vi "Dashboard custom_bartender&global&gripper&camera3.vi"() -> ()   [LabVIEW 2017]
uses:
  C:/Users/IMR Lab/Documents/LabVIEW Data/UniversalRobotsSDK_LABView/LabVIEW/Examples/LabVIEW10/UnderAutomation.UniversalRobots.dll
  UnderAutomation.UniversalRobots.dll
  Global 1.vi
panel:
  out "3rd Order":bool
  out "2nd Order":bool
  out "1st Order":bool
  out "Rx":dbl
  out "Rz":dbl
  out "Ry":dbl
  out "Enabled":bool
  out "Port":i32
  in  "Move to particular posture":bool
  in  "Move to Zero position":bool
  out "Connected":bool
  in  "Robot IP(192.168.112.182)":string
  out "Connect error":errorcluster
  in  "Power on\nRelease brake":bool
  in  "Power off":bool
  in  "Connect":bool
  in  "Send script":bool
  in  "Script to execute":string
  out "Powered on":bool
  out "X":dbl
  out "Y":dbl
  out "Z":dbl
  out "License state":string
  # "e"
  # "movej( get_inverse_kin(p[0.3138, 0.0814, 0.1647, 0.4226, -2.3876, -2.3851]),  a=0.5, v=0.25, t=0, r=0)"
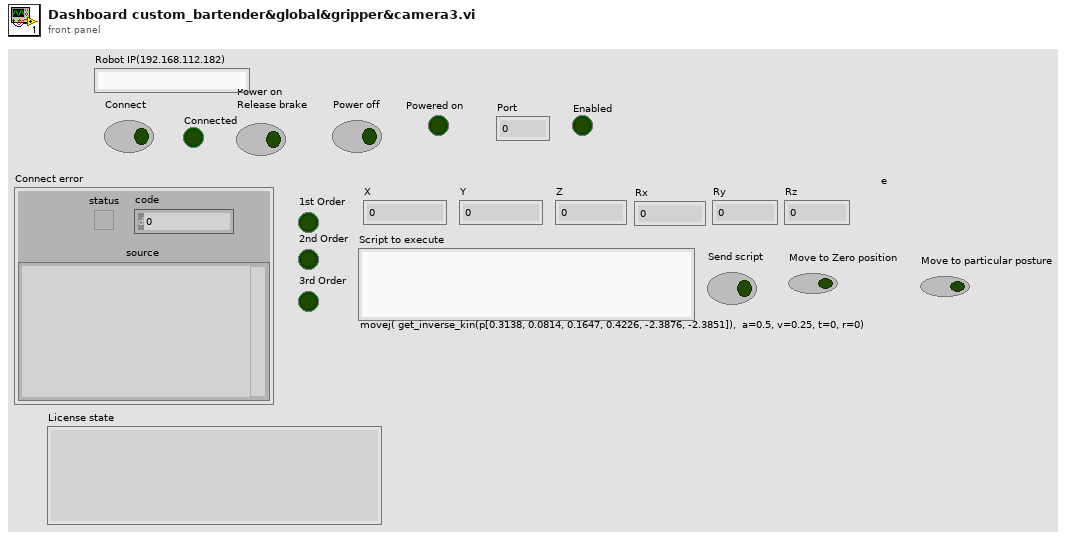
[diagram p1: front panel]
types:
  T1 = enum16{"Standard", "Buffered", "CRLF", "Immediate"}
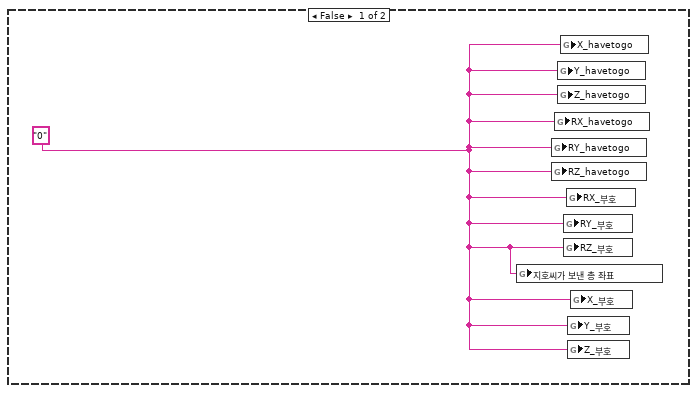
[diagram p2: hidden frame]
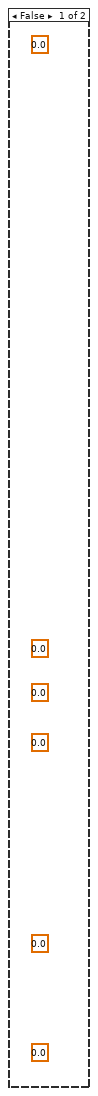
[diagram p3: hidden frame]
diagram:
  w2 = ""
  # "미니콜라 따르는 자세"
  # "술잔 중간지점 가는 자세"
  # "짐빔에서 토닉이동 준비 자세"
  # "술잔 따르는 자세2"
  # "술잔 위로 가는 자세2"
  # "토닉워터 뺴는 자세"
  # "토닉워 들어올리는 자세"
  # "토닉워터 가는 자세"
  # "토닉워터 보는 자세"
  # "짐빔 들어올리는 자세"
  # "짐빔로 가는 자세"
  # "짐빔 보는 자세"
  # "콜라 뺴는 자세"
  # "콜라 들어올리는 자세"
  # "콜라로 가는 자세"
  # "콜라 보는 자세"
  # "술잔 따르는 자세"
  # "술잔 위로 가는 자세"
  # "잭다니엘 들어올리는 자세"
  # "잭다니엘 위치로 가는 자세"
  # "잭다니엘 보는 자세"
  # "1자로 서는 자세"
  # "Example : Display power on status"
  # "Create a UR\ncobot instance"
  # "Show license state"
  # "Register your confidential license key to exit\ntrial period and use this library forever"
  # "Power off when button is clicked"
  # "Power on and release brake when button is clicked"
  # "Get your UR Dashboard interface"
  n1 = global write "Global 1.vi" "TCP 스위치"(FALSE ("TCP 스위치")) -> ()
  n2 = global write "Global 1.vi" "미니콜라 따르는 자세"("movej([-0.0902,-1.8120,-1.9241,-3.5769,6.2827,8.4658], a=0.5, v=0.25, t=0, r=0)") -> ()
  n3 = global write "Global 1.vi" "잭다니엘 들어올리는 자세"("movej([0.8116,-2.0223,-1.2828,-3.0107,4.3284,5.9341], a=0.5, v=0.25, t=0, r=0)") -> ()
  n4 = global write "Global 1.vi" "짐빔 토닉 이동 준비자세"("movej([-0.5421,-0.8131,0.8439,-0.0538,2.5052,5.9032], a=0.5, v=0.25, t=0, r=0)") -> ()
  n5 = global write "Global 1.vi" "토닉 빼는 자세"("movej([-0.5277,-1.5104,1.5889,-0.0548,2.5728,5.9025], a=0.5, v=0.25, t=0, r=0)") -> ()
  n6 = global write "Global 1.vi" "잭다닐 위치로 가는 자세"("movej([0.8116,-2.3119,-1.606,-2.3958,4.3284,5.9341], a=0.5, v=0.25, t=0, r=0)") -> ()
  n7 = global write "Global 1.vi" "토닉 드는 자세"("movej([-1.0311,-1.1460,1.5830,-0.4348,2.0708,5.9048], a=0.5, v=0.25, t=0, r=0)") -> ()
  n8 = global write "Global 1.vi" "토닉 보는 자세"("movej([-0.4690,-1.1292,2.1508,-1.0119,2.6124,5.9032], a=0.5, v=0.25, t=0, r=0)") -> ()
  n9 = global write "Global 1.vi" "술잔 위로 가는 자세 2"("movej([0.0485,-1.6015,2.5780,-1.0382,-0.0520,5.3649], a=0.5, v=0.25, t=0, r=0)") -> ()
  n10 = global write "Global 1.vi" "1자로 서는 자세"("movej([3.1412,-1.5708,0,-1.5708,3.1412,5.8904], a=0.5, v=0.25, t=0, r=0)") -> ()
  n11 = global write "Global 1.vi" "짐빔 들어올리는 자세"("movej([-0.5421,-0.8131,0.8439,-0.0538,2.5052,5.9032], a=0.5, v=0.25, t=0, r=0)") -> ()
  n12 = global write "Global 1.vi" "술잔 위로 가는 자세"("movej([-0.0903,-2.0548,-2.0169,-3.3289,6.2826,7.4091], a=0.5, v=0.25, t=0, r=0)") -> ()
  n13 = global write "Global 1.vi" "토닉 가는자세"("movej([-0.9924,-0.8742,1.7459,-0.8837,2.0958,5.9048], a=0.5, v=0.25, t=0, r=0)") -> ()
  n14 = global write "Global 1.vi" "잭다니엘 보는 자세"("movej([0,-2.2170,-1.4226,-2.2842,3.1412,6.2832], a=0.5, v=0.25, t=0, r=0)") -> ()
  n15 = global write "Global 1.vi" "짐빔 위치로 가는 자세"("movej([-0.5436,-0.4519,0.8428,-0.3534,2.6134,5.9032], a=0.5, v=0.25, t=0, r=0)") -> ()
  n16 = global write "Global 1.vi" "콜라 보는 자세"("movej([0,-1.8110,-2.1684,-2.3033,3.1543,5.9213], a=0.5, v=0.25, t=0, r=0)") -> ()
  n17 = global write "Global 1.vi" "콜라로 가는자세"("movej([1.2020,-2.166,-1.9385,-2.1863,4.3172,5.9210], a=0.5, v=0.25, t=0, r=0)") -> ()
  n18 = global write "Global 1.vi" "콜라 빼는 자세"("movej([0.8789,-1.5237,-2.1070,-2.6679, 3.9917,5.9085], a=0.5, v=0.25, t=0, r=0)") -> ()
  n19 = global write "Global 1.vi" "콜라 드는 자세"("movej([1.2020,-1.8452,-1.7403,-2.7082,4.3162,5.9158], a=0.5, v=0.25, t=0, r=0)") -> ()
  n20 = global write "Global 1.vi" "술 따르는 자세 2"("movej([0.0412,-1.9708,2.4700,-1.0157,-0.0618,4.8998], a=0.5, v=0.25, t=0, r=0)") -> ()
  n21 = global write "Global 1.vi" "잭다니엘 카메라 값"(w2) -> ()
  n22 = global write "Global 1.vi" "술 따르는 자세"("movej([-0.0902,-1.9024,-1.9241,-3.5769,6.2827,8.4692], a=0.5, v=0.25, t=0, r=0)") -> ()
  n23 = global write "Global 1.vi" "짐빔 보는 자세"("movej([-0.0364,-0.6154,0.9421,-0.3291,3.1047,5.9020], a=0.5, v=0.25, t=0, r=0)") -> ()
  n24 = global write "Global 1.vi" "콜라 카메라 값"(w2) -> ()
  n25 = global write "Global 1.vi" "토닉 카메라 값"(w2) -> ()
  n26 = global write "Global 1.vi" "짐빔 카메라 값"(w2) -> ()
  n27 = constructor class="UR"() -> (reference out=w28:refnum<k24>)  [unwired: 3 in, 2 out]
  n28 = global write "Global 1.vi" "술잔 중간지점"("movej([-0.2173,-1.9485,-1.6874,-3.9352,6.2671,7.2276], a=0.5, v=0.25, t=0, r=0)") -> ()
  n29 = while {
    tunnel: w28 -> [w34]
    stop <- FALSE stop-if-true
    # "Connect to the robot when button is pressed"
    # "Show if primary interface is connected"
    # "Get your UR primary interface"
    n30 = property class="UR"(reference=w34) -> ("PrimaryInterface"=w37:refnum<k24>)  [unwired: 1 in, 2 out]
    n31 = Wait (ms)(milliseconds to wait=u32 50) -> ()  [unwired: 1 out]
    n32 = property class="PrimaryInterfaceClientInternal"(reference=w37) -> ("Connected"=w36:bool)  [unwired: 1 in, 2 out]
    "Connected" <- w36
    n33 = case shown="True" "Connect" {
      tunnel: w34 -> [_ w1120]
      frame False {
      }
      frame True {
        n34 = flat-sequence {
          tunnel: w1120 -> [w1122]
          frame #0 {
            n35 = invoke class="UR" method="Connect"(reference=w1122, "ip"="Robot IP(192.168.112.182)") -> (error out=→"Connect error":errorcluster)  [unwired: 2 in, 3 out]
          }
        }
      }
    }
    n36 = case shown="True" w36 {
      tunnel: w37 -> [_ w50]
      frame False {
        (unwired) 0.0 ("Rx")
        (unwired) 0.0 ("Rz")
        (unwired) 0.0 ("Ry")
        (unwired) 0.0 ("Z")
        (unwired) 0.0 ("X")
        (unwired) 0.0 ("Y")
      }
      frame True {
        # "Send URScript when button pressed"
        # "Example : Display current cartesian pose"
        n37 = property class="PrimaryInterfaceClientInternal"(reference=w50) -> ("Script"=w51:refnum<k24>)  [unwired: 1 in, 2 out]
        n38 = global read "Global 1.vi" "2nd Order"() -> (w54:bool)
        "2nd Order" <- w54
        n39 = global read "Global 1.vi" "3rd Order"() -> (w53:bool)
        "3rd Order" <- w53
        n40 = global read "Global 1.vi" "1st Order"() -> (w55:bool)
        "1st Order" <- w55
        n41 = Build Array(w55, w54, w53) -> (w56:bool[])
        n42 = Boolean Array To Number(Boolean array=w56) -> (number=w52:u32)
        n43 = case shown="100" w52 {
          tunnel: w51 -> [_ w107 w434 _ w764 _ _ _]
          frame 0, Default {
          }
          frame 1 {
            # "잭다 : 콜라 = 1 : 3"
            # "1st order"
            n44 = flat-sequence {
              tunnel: w107 -> [w111]
              tunnel: [w110] -> w106
              tunnel: w106 -> [w115]
              tunnel: [w113] -> w100
              tunnel: w100 -> [w118]
              tunnel: [w118] -> w98
              tunnel: w98 -> [w121]
              tunnel: [w121] -> w76
              tunnel: w76 -> [w125]
              tunnel: [w125] -> w73
              tunnel: w73 -> [w132]
              tunnel: [w132] -> w72
              tunnel: w72 -> [w208]
              tunnel: [w208] -> w75
              tunnel: w75 -> [w211]
              tunnel: [w211] -> w74
              tunnel: w74 -> [w215]
              tunnel: [w212] -> w99
              tunnel: w99 -> [w218]
              tunnel: [w218] -> w97
              tunnel: w97 -> [w221]
              tunnel: [w221] -> w96
              tunnel: w96 -> [w223]
              tunnel: [w222] -> w84
              tunnel: w84 -> [w227]
              tunnel: [w226] -> w83
              tunnel: w83 -> [w231]
              tunnel: [w230] -> w105
              tunnel: w105 -> [w236]
              tunnel: [w234] -> w104
              tunnel: w104 -> [w239]
              tunnel: [w238] -> w82
              tunnel: w82 -> [w243]
              tunnel: [w242] -> w81
              tunnel: [w246] -> w71
              tunnel: w81 -> [w248]
              tunnel: [w250] -> w95
              tunnel: w71 -> [w251]
              tunnel: w95 -> [w256]
              tunnel: [w256] -> w94
              tunnel: w94 -> [w259]
              tunnel: [w259] -> w93
              tunnel: w93 -> [w261]
              tunnel: [w260] -> w69
              tunnel: w69 -> [w267]
              tunnel: [w267] -> w68
              tunnel: w68 -> [w274]
              tunnel: [w274] -> w67
              tunnel: w67 -> [w350]
              tunnel: [w350] -> w66
              tunnel: w66 -> [w353]
              tunnel: [w353] -> w65
              tunnel: [w354] -> w92
              tunnel: w65 -> [w355]
              tunnel: w92 -> [w360]
              tunnel: [w360] -> w91
              tunnel: w91 -> [w363]
              tunnel: [w363] -> w70
              tunnel: [w364] -> w90
              tunnel: w70 -> [w365]
              tunnel: w90 -> [w369]
              tunnel: [w368] -> w80
              tunnel: w80 -> [w373]
              tunnel: [w372] -> w79
              tunnel: w79 -> [w377]
              tunnel: [w376] -> w103
              tunnel: w103 -> [w381]
              tunnel: [w380] -> w102
              tunnel: w102 -> [w385]
              tunnel: [w384] -> w78
              tunnel: w78 -> [w389]
              tunnel: [w388] -> w77
              tunnel: w77 -> [w393]
              tunnel: [w392] -> w89
              tunnel: w89 -> [w397]
              tunnel: [w396] -> w101
              tunnel: w101 -> [w401]
              tunnel: [w400] -> w87
              tunnel: [w404] -> w88
              tunnel: w87 -> [w404]
              tunnel: [w407] -> w86
              tunnel: w88 -> [w407]
              tunnel: w86 -> [w411]
              tunnel: [w410] -> w85
              tunnel: w85 -> [w414]
              frame #0 {
                # "초기자세"
                n45 = global read "Global 1.vi" "1자로 서는 자세"() -> (w109:string)
                n46 = invoke class="PrimaryInterfaceScript" method="Send"(reference=w111, "script"=w109) -> (reference out=w110:refnum<k24>)  [unwired: 2 in, 3 out]
                n47 = Wait (ms)(milliseconds to wait=u32 15000) -> ()  [unwired: 1 out]
              }
              frame #1 {
                # "잭다니엘 보기"
                n48 = global read "Global 1.vi" "잭다니엘 보는 자세"() -> (w114:string)
                n49 = invoke class="PrimaryInterfaceScript" method="Send"(reference=w115, "script"=w114) -> (reference out=w113:refnum<k24>)  [unwired: 2 in, 3 out]
                n50 = Wait (ms)(milliseconds to wait=u32 15000) -> ()  [unwired: 1 out]
              }
              frame #2 {
                # "그리퍼 열기"
                n51 = global write "Global 1.vi" "그리퍼 열림"(TRUE ("그리퍼 열림")) -> ()
                n52 = Wait (ms)(milliseconds to wait=u32 300) -> ()  [unwired: 1 out]
              }
              frame #3 {
                n53 = global write "Global 1.vi" "그리퍼 열림"(FALSE ("그리퍼 열림")) -> ()
                n54 = Wait (ms)(milliseconds to wait=u32 300) -> ()  [unwired: 1 out]
              }
              frame #4 {
                # "tcp 키는 스위치 보단\n파이썬한테 \n값 보내달라하는\n요청 보내는 걸로 \n바꾸기"
                n55 = global write "Global 1.vi" "몇번 병을 볼것인가"("0" ("몇번 병을 볼것인가")) -> ()
                n56 = global write "Global 1.vi" "TCP 스위치"(TRUE ("그리퍼 열림")) -> ()
                n57 = Wait Until Next ms Multiple(millisecond multiple=u32 500 ("milliseconds to wait")) -> ()  [unwired: 1 out]
              }
              frame #5 {
                n58 = global read "Global 1.vi" "X_부호"() -> (w128:string)
                n59 = global read "Global 1.vi" "Z_부호"() -> (w126:string)
                n60 = global read "Global 1.vi" "Y_부호"() -> (w127:string)
                n61 = case shown="\"1\"" w126 {
                  frame "False", Default {
                  }
                  frame "True" {
                  }
                  frame "2" {
                  }
                  frame "1" {
                    n62 = global read "Global 1.vi" "Z_havetogo"() -> (w134:string)
                    n63 = Decimal String To Number(string=w134) -> (number=w137:i32)  [unwired: 2 in, 1 out]
                    n64 = To Double Precision Float(number=w137) -> (double precision float=w136:dbl)
                    n65 = Format Into String(format string="-%f", w136) -> (resulting string=w133:string)  [unwired: 2 in, 1 out]
                    n66 = global write "Global 1.vi" "Z_havetogo"(w133) -> ()
                  }
                }
                n67 = case shown="\"1\"" w127 {
                  frame "False", Default {
                  }
                  frame "True" {
                  }
                  frame "2" {
                  }
                  frame "1" {
                    n68 = global read "Global 1.vi" "Y_havetogo"() -> (w139:string)
                    n69 = Decimal String To Number(string=w139) -> (number=w142:i32)  [unwired: 2 in, 1 out]
                    n70 = To Double Precision Float(number=w142) -> (double precision float=w140:dbl)
                    n71 = Format Into String(format string="-%f", w140) -> (resulting string=w138:string)  [unwired: 2 in, 1 out]
                    n72 = global write "Global 1.vi" "Y_havetogo"(w138) -> ()
                  }
                }
                n73 = case shown="\"1\"" w128 {
                  frame "False", Default {
                  }
                  frame "True" {
                  }
                  frame "2" {
                  }
                  frame "1" {
                    n74 = global read "Global 1.vi" "X_havetogo"() -> (w144:string)
                    n75 = Decimal String To Number(string=w144) -> (number=w147:i32)  [unwired: 2 in, 1 out]
                    n76 = To Double Precision Float(number=w147) -> (double precision float=w146:dbl)
                    n77 = Format Into String(format string="-%f", w146) -> (resulting string=w143:string)  [unwired: 2 in, 1 out]
                    n78 = global write "Global 1.vi" "X_havetogo"(w143) -> ()
                  }
                }
                n79 = global read "Global 1.vi" "RX_부호"() -> (w131:string)
                n80 = global read "Global 1.vi" "RZ_부호"() -> (w129:string)
                n81 = global read "Global 1.vi" "RY_부호"() -> (w130:string)
                n82 = case shown="\"1\"" w129 {
                  frame "False", Default {
                  }
                  frame "True" {
                  }
                  frame "2" {
                  }
                  frame "1" {
                    n83 = global read "Global 1.vi" "RZ_havetogo"() -> (w149:string)
                    n84 = Decimal String To Number(string=w149) -> (number=w152:i32)  [unwired: 2 in, 1 out]
                    n85 = To Double Precision Float(number=w152) -> (double precision float=w151:dbl)
                    n86 = Format Into String(format string="-%f", w151) -> (resulting string=w148:string)  [unwired: 2 in, 1 out]
                    n87 = global write "Global 1.vi" "RZ_havetogo"(w148) -> ()
                  }
                }
                n88 = case shown="\"1\"" w130 {
                  frame "False", Default {
                  }
                  frame "True" {
                  }
                  frame "2" {
                  }
                  frame "1" {
                    n89 = global read "Global 1.vi" "RY_havetogo"() -> (w154:string)
                    n90 = Decimal String To Number(string=w154) -> (number=w157:i32)  [unwired: 2 in, 1 out]
                    n91 = To Double Precision Float(number=w157) -> (double precision float=w155:dbl)
                    n92 = Format Into String(format string="-%f", w155) -> (resulting string=w153:string)  [unwired: 2 in, 1 out]
                    n93 = global write "Global 1.vi" "RY_havetogo"(w153) -> ()
                  }
                }
                n94 = case shown="\"1\"" w131 {
                  frame "False", Default {
                  }
                  frame "True" {
                  }
                  frame "2" {
                  }
                  frame "1" {
                    n95 = global read "Global 1.vi" "RX_havetogo"() -> (w159:string)
                    n96 = Decimal String To Number(string=w159) -> (number=w162:i32)  [unwired: 2 in, 1 out]
                    n97 = To Double Precision Float(number=w162) -> (double precision float=w161:dbl)
                    n98 = Format Into String(format string="-%f", w161) -> (resulting string=w158:string)  [unwired: 2 in, 1 out]
                    n99 = global write "Global 1.vi" "RX_havetogo"(w158) -> ()
                  }
                }
              }
              frame #6 {
                n100 = global read "Global 1.vi" "X_havetogo"() -> (w174:string)
                n101 = global read "Global 1.vi" "Y_havetogo"() -> (w173:string)
                n102 = global read "Global 1.vi" "Z_havetogo"() -> (w172:string)
                n103 = global read "Global 1.vi" "RX_havetogo"() -> (w171:string)
                n104 = global read "Global 1.vi" "RY_havetogo"() -> (w170:string)
                n105 = global read "Global 1.vi" "RZ_havetogo"() -> (w169:string)
                n106 = Decimal String To Number(string=w172) -> (number=w198:i32)  [unwired: 2 in, 1 out]
                n107 = Decimal String To Number(string=w174) -> (number=w204:i32)  [unwired: 2 in, 1 out]
                n108 = Decimal String To Number(string=w173) -> (number=w201:i32)  [unwired: 2 in, 1 out]
                n109 = Decimal String To Number(string=w171) -> (number=w195:i32)  [unwired: 2 in, 1 out]
                n110 = Decimal String To Number(string=w170) -> (number=w192:i32)  [unwired: 2 in, 1 out]
                n111 = Decimal String To Number(string=w169) -> (number=w189:i32)  [unwired: 2 in, 1 out]
                n112 = To Double Precision Float(number=w198) -> (double precision float=w200:dbl)
                n113 = To Double Precision Float(number=w204) -> (double precision float=w206:dbl)
                n114 = To Double Precision Float(number=w201) -> (double precision float=w203:dbl)
                n115 = To Double Precision Float(number=w195) -> (double precision float=w197:dbl)
                n116 = To Double Precision Float(number=w192) -> (double precision float=w194:dbl)
                n117 = Multiply(x=w206, y=0.001) -> (x*y=w188:dbl)
                n118 = Multiply(x=w200, y=0.001) -> (x*y=w184:dbl)
                n119 = Multiply(x=w203, y=0.001) -> (x*y=w186:dbl)
                n120 = Multiply(x=w197, y=0.001) -> (x*y=w182:dbl)
                n121 = global read "Global 1.vi" "x"() -> (w168:dbl)
                n122 = Multiply(x=w194, y=0.001) -> (x*y=w180:dbl)
                n123 = global read "Global 1.vi" "y"() -> (w167:dbl)
                n124 = global read "Global 1.vi" "rx"() -> (w165:dbl)
                n125 = global read "Global 1.vi" "z"() -> (w166:dbl)
                n126 = To Double Precision Float(number=w189) -> (double precision float=w191:dbl)
                n127 = Add(x=w168, y=w188) -> (x+y=w187:dbl)
                n128 = Multiply(x=w191, y=0.001) -> (x*y=w178:dbl)
                n129 = Add(x=w184, y=w166) -> (x+y=w183:dbl)
                n130 = Add(x=w186, y=w167) -> (x+y=w185:dbl)
                n131 = global read "Global 1.vi" "ry"() -> (w163:dbl)
                n132 = global read "Global 1.vi" "rz"() -> (w164:dbl)
                n133 = Add(x=w182, y=w165) -> (x+y=w181:dbl)
                n134 = Add(x=w180, y=w163) -> (x+y=w179:dbl)
                n135 = Add(x=w178, y=w164) -> (x+y=w177:dbl)
                n136 = Format Into String(format string="movej( get_inverse_kin(p[%f, %f, %f, %f, %f, %f]), a= 0.5, v=0.25, t=0, r=0)", w187, w185, w183, w181, w179, w177) -> (resulting string=w175:string)  [unwired: 2 in, 1 out]
                n137 = global write "Global 1.vi" "잭다니엘 카메라 값"(w175) -> ()
                n138 = Wait (ms)(milliseconds to wait=u32 300) -> ()  [unwired: 1 out]
              }
              frame #7 {
                n139 = global write "Global 1.vi" "TCP 스위치"(FALSE ("그리퍼 열림")) -> ()
                n140 = Wait Until Next ms Multiple(millisecond multiple=u32 300 ("milliseconds to wait")) -> ()  [unwired: 1 out]
              }
              frame #8 {
                # "잭다니엘 위치로 가기"
                n141 = global read "Global 1.vi" "잭다니엘 카메라 값"() -> (w214:string)
                n142 = invoke class="PrimaryInterfaceScript" method="Send"(reference=w215, "script"=w214) -> (reference out=w212:refnum<k24>)  [unwired: 2 in, 3 out]
                n143 = Wait (ms)(milliseconds to wait=u32 7000) -> ()  [unwired: 1 out]
              }
              frame #9 {
                # "그리퍼 닫기"
                n144 = global write "Global 1.vi" "그리퍼 닫힘"(TRUE ("그리퍼 열림")) -> ()
                n145 = Wait (ms)(milliseconds to wait=u32 300) -> ()  [unwired: 1 out]
              }
              frame #10 {
                n146 = global write "Global 1.vi" "그리퍼 닫힘"(FALSE ("그리퍼 열림")) -> ()
                n147 = Wait (ms)(milliseconds to wait=u32 3000) -> ()  [unwired: 1 out]
              }
              frame #11 {
                # "잭다니엘 들기"
                n148 = global read "Global 1.vi" "잭다니엘 들어올리는 자세"() -> (w225:string)
                n149 = invoke class="PrimaryInterfaceScript" method="Send"(reference=w223, "script"=w225) -> (reference out=w222:refnum<k24>)  [unwired: 2 in, 3 out]
                n150 = Wait (ms)(milliseconds to wait=u32 5000) -> ()  [unwired: 1 out]
              }
              frame #12 {
                # "술잔 중간지점으로 이동"
                n151 = global read "Global 1.vi" "술잔 중간지점"() -> (w228:string)
                n152 = invoke class="PrimaryInterfaceScript" method="Send"(reference=w227, "script"=w228) -> (reference out=w226:refnum<k24>)  [unwired: 2 in, 3 out]
                n153 = Wait (ms)(milliseconds to wait=u32 15000) -> ()  [unwired: 1 out]
              }
              frame #13 {
                # "술잔 쪽으로 이동"
                n154 = global read "Global 1.vi" "술잔 위로 가는 자세"() -> (w232:string)
                n155 = invoke class="PrimaryInterfaceScript" method="Send"(reference=w231, "script"=w232) -> (reference out=w230:refnum<k24>)  [unwired: 2 in, 3 out]
                n156 = Wait (ms)(milliseconds to wait=u32 5000) -> ()  [unwired: 1 out]
              }
              frame #14 {
                # "술따르기"
                n157 = global read "Global 1.vi" "술 따르는 자세"() -> (w235:string)
                n158 = invoke class="PrimaryInterfaceScript" method="Send"(reference=w236, "script"=w235) -> (reference out=w234:refnum<k24>)  [unwired: 2 in, 3 out]
                n159 = Wait (ms)(milliseconds to wait=u32 9000) -> ()  [unwired: 1 out]
              }
              frame #15 {
                # "술따르기 중단"
                n160 = global read "Global 1.vi" "술잔 위로 가는 자세"() -> (w240:string)
                n161 = invoke class="PrimaryInterfaceScript" method="Send"(reference=w239, "script"=w240) -> (reference out=w238:refnum<k24>)  [unwired: 2 in, 3 out]
                n162 = Wait (ms)(milliseconds to wait=u32 4000) -> ()  [unwired: 1 out]
              }
              frame #16 {
                # "술잔 중간지점으로 이동"
                n163 = global read "Global 1.vi" "술잔 중간지점"() -> (w244:string)
                n164 = invoke class="PrimaryInterfaceScript" method="Send"(reference=w243, "script"=w244) -> (reference out=w242:refnum<k24>)  [unwired: 2 in, 3 out]
                n165 = Wait (ms)(milliseconds to wait=u32 7000) -> ()  [unwired: 1 out]
              }
              frame #17 {
                # "잭다니엘 들었던 곳으로"
                n166 = global read "Global 1.vi" "잭다니엘 들어올리는 자세"() -> (w247:string)
                n167 = invoke class="PrimaryInterfaceScript" method="Send"(reference=w248, "script"=w247) -> (reference out=w246:refnum<k24>)  [unwired: 2 in, 3 out]
                n168 = Wait (ms)(milliseconds to wait=u32 10000) -> ()  [unwired: 1 out]
              }
              frame #18 {
                # "잭다니엘 내려놓기"
                n169 = global read "Global 1.vi" "잭다닐 위치로 가는 자세"() -> (w253:string)
                n170 = invoke class="PrimaryInterfaceScript" method="Send"(reference=w251, "script"=w253) -> (reference out=w250:refnum<k24>)  [unwired: 2 in, 3 out]
                n171 = Wait (ms)(milliseconds to wait=u32 5000) -> ()  [unwired: 1 out]
              }
              frame #19 {
                # "그리퍼 열기"
                n172 = global write "Global 1.vi" "그리퍼 열림"(TRUE ("그리퍼 열림")) -> ()
                n173 = Wait (ms)(milliseconds to wait=u32 300) -> ()  [unwired: 1 out]
              }
              frame #20 {
                n174 = global write "Global 1.vi" "그리퍼 열림"(FALSE ("그리퍼 열림")) -> ()
                n175 = Wait (ms)(milliseconds to wait=u32 3000) -> ()  [unwired: 1 out]
              }
              frame #21 {
                # "콜라보러가기"
                n176 = global read "Global 1.vi" "콜라 보는 자세"() -> (w263:string)
                n177 = invoke class="PrimaryInterfaceScript" method="Send"(reference=w261, "script"=w263) -> (reference out=w260:refnum<k24>)  [unwired: 2 in, 3 out]
                n178 = Wait (ms)(milliseconds to wait=u32 8000) -> ()  [unwired: 1 out]
              }
              frame #22 {
                # "tcp 키는 스위치 보단\n파이썬한테 \n값 보내달라하는\n요청 보내는 걸로 \n바꾸기"
                n179 = global write "Global 1.vi" "몇번 병을 볼것인가"("1" ("몇번 병을 볼것인가")) -> ()
                n180 = global write "Global 1.vi" "TCP 스위치"(TRUE ("그리퍼 열림")) -> ()
                n181 = Wait Until Next ms Multiple(millisecond multiple=u32 500 ("milliseconds to wait")) -> ()  [unwired: 1 out]
              }
              frame #23 {
                n182 = global read "Global 1.vi" "X_부호"() -> (w270:string)
                n183 = global read "Global 1.vi" "Z_부호"() -> (w268:string)
                n184 = global read "Global 1.vi" "Y_부호"() -> (w269:string)
                n185 = case shown="\"1\"" w268 {
                  frame "False", Default {
                  }
                  frame "True" {
                  }
                  frame "2" {
                  }
                  frame "1" {
                    n186 = global read "Global 1.vi" "Z_havetogo"() -> (w276:string)
                    n187 = Decimal String To Number(string=w276) -> (number=w279:i32)  [unwired: 2 in, 1 out]
                    n188 = To Double Precision Float(number=w279) -> (double precision float=w278:dbl)
                    n189 = Format Into String(format string="-%f", w278) -> (resulting string=w275:string)  [unwired: 2 in, 1 out]
                    n190 = global write "Global 1.vi" "Z_havetogo"(w275) -> ()
                  }
                }
                n191 = case shown="\"1\"" w269 {
                  frame "False", Default {
                  }
                  frame "True" {
                  }
                  frame "2" {
                  }
                  frame "1" {
                    n192 = global read "Global 1.vi" "Y_havetogo"() -> (w281:string)
                    n193 = Decimal String To Number(string=w281) -> (number=w284:i32)  [unwired: 2 in, 1 out]
                    n194 = To Double Precision Float(number=w284) -> (double precision float=w282:dbl)
                    n195 = Format Into String(format string="-%f", w282) -> (resulting string=w280:string)  [unwired: 2 in, 1 out]
                    n196 = global write "Global 1.vi" "Y_havetogo"(w280) -> ()
                  }
                }
                n197 = case shown="\"1\"" w270 {
                  frame "False", Default {
                  }
                  frame "True" {
                  }
                  frame "2" {
                  }
                  frame "1" {
                    n198 = global read "Global 1.vi" "X_havetogo"() -> (w286:string)
                    n199 = Decimal String To Number(string=w286) -> (number=w289:i32)  [unwired: 2 in, 1 out]
                    n200 = To Double Precision Float(number=w289) -> (double precision float=w288:dbl)
                    n201 = Format Into String(format string="-%f", w288) -> (resulting string=w285:string)  [unwired: 2 in, 1 out]
                    n202 = global write "Global 1.vi" "X_havetogo"(w285) -> ()
                  }
                }
                n203 = global read "Global 1.vi" "RX_부호"() -> (w273:string)
                n204 = global read "Global 1.vi" "RZ_부호"() -> (w271:string)
                n205 = global read "Global 1.vi" "RY_부호"() -> (w272:string)
                n206 = case shown="\"1\"" w271 {
                  frame "False", Default {
                  }
                  frame "True" {
                  }
                  frame "2" {
                  }
                  frame "1" {
                    n207 = global read "Global 1.vi" "RZ_havetogo"() -> (w291:string)
                    n208 = Decimal String To Number(string=w291) -> (number=w294:i32)  [unwired: 2 in, 1 out]
                    n209 = To Double Precision Float(number=w294) -> (double precision float=w293:dbl)
                    n210 = Format Into String(format string="-%f", w293) -> (resulting string=w290:string)  [unwired: 2 in, 1 out]
                    n211 = global write "Global 1.vi" "RZ_havetogo"(w290) -> ()
                  }
                }
                n212 = case shown="\"1\"" w272 {
                  frame "False", Default {
                  }
                  frame "True" {
                  }
                  frame "2" {
                  }
                  frame "1" {
                    n213 = global read "Global 1.vi" "RY_havetogo"() -> (w296:string)
                    n214 = Decimal String To Number(string=w296) -> (number=w299:i32)  [unwired: 2 in, 1 out]
                    n215 = To Double Precision Float(number=w299) -> (double precision float=w297:dbl)
                    n216 = Format Into String(format string="-%f", w297) -> (resulting string=w295:string)  [unwired: 2 in, 1 out]
                    n217 = global write "Global 1.vi" "RY_havetogo"(w295) -> ()
                  }
                }
                n218 = case shown="\"1\"" w273 {
                  frame "False", Default {
                  }
                  frame "True" {
                  }
                  frame "2" {
                  }
                  frame "1" {
                    n219 = global read "Global 1.vi" "RX_havetogo"() -> (w301:string)
                    n220 = Decimal String To Number(string=w301) -> (number=w304:i32)  [unwired: 2 in, 1 out]
                    n221 = To Double Precision Float(number=w304) -> (double precision float=w303:dbl)
                    n222 = Format Into String(format string="-%f", w303) -> (resulting string=w300:string)  [unwired: 2 in, 1 out]
                    n223 = global write "Global 1.vi" "RX_havetogo"(w300) -> ()
                  }
                }
              }
              frame #24 {
                n224 = global read "Global 1.vi" "X_havetogo"() -> (w316:string)
                n225 = global read "Global 1.vi" "Y_havetogo"() -> (w315:string)
                n226 = global read "Global 1.vi" "Z_havetogo"() -> (w314:string)
                n227 = global read "Global 1.vi" "RX_havetogo"() -> (w313:string)
                n228 = global read "Global 1.vi" "RY_havetogo"() -> (w312:string)
                n229 = global read "Global 1.vi" "RZ_havetogo"() -> (w311:string)
                n230 = Decimal String To Number(string=w314) -> (number=w340:i32)  [unwired: 2 in, 1 out]
                n231 = Decimal String To Number(string=w316) -> (number=w346:i32)  [unwired: 2 in, 1 out]
                n232 = Decimal String To Number(string=w315) -> (number=w343:i32)  [unwired: 2 in, 1 out]
                n233 = Decimal String To Number(string=w313) -> (number=w337:i32)  [unwired: 2 in, 1 out]
                n234 = Decimal String To Number(string=w312) -> (number=w334:i32)  [unwired: 2 in, 1 out]
                n235 = Decimal String To Number(string=w311) -> (number=w331:i32)  [unwired: 2 in, 1 out]
                n236 = To Double Precision Float(number=w340) -> (double precision float=w342:dbl)
                n237 = To Double Precision Float(number=w346) -> (double precision float=w348:dbl)
                n238 = To Double Precision Float(number=w343) -> (double precision float=w345:dbl)
                n239 = To Double Precision Float(number=w337) -> (double precision float=w339:dbl)
                n240 = To Double Precision Float(number=w334) -> (double precision float=w336:dbl)
                n241 = Multiply(x=w348, y=0.001) -> (x*y=w330:dbl)
                n242 = Multiply(x=w342, y=0.001) -> (x*y=w326:dbl)
                n243 = Multiply(x=w345, y=0.001) -> (x*y=w328:dbl)
                n244 = Multiply(x=w339, y=0.001) -> (x*y=w324:dbl)
                n245 = global read "Global 1.vi" "x"() -> (w310:dbl)
                n246 = Multiply(x=w336, y=0.001) -> (x*y=w322:dbl)
                n247 = global read "Global 1.vi" "y"() -> (w309:dbl)
                n248 = global read "Global 1.vi" "rx"() -> (w307:dbl)
                n249 = global read "Global 1.vi" "z"() -> (w308:dbl)
                n250 = To Double Precision Float(number=w331) -> (double precision float=w333:dbl)
                n251 = Add(x=w310, y=w330) -> (x+y=w329:dbl)
                n252 = Multiply(x=w333, y=0.001) -> (x*y=w320:dbl)
                n253 = Add(x=w326, y=w308) -> (x+y=w325:dbl)
                n254 = Add(x=w328, y=w309) -> (x+y=w327:dbl)
                n255 = global read "Global 1.vi" "ry"() -> (w305:dbl)
                n256 = global read "Global 1.vi" "rz"() -> (w306:dbl)
                n257 = Add(x=w324, y=w307) -> (x+y=w323:dbl)
                n258 = Add(x=w322, y=w305) -> (x+y=w321:dbl)
                n259 = Add(x=w320, y=w306) -> (x+y=w319:dbl)
                n260 = Format Into String(format string="movej( get_inverse_kin(p[%f, %f, %f, %f, %f, %f]), a= 0.5, v=0.25, t=0, r=0)", w329, w327, w325, w323, w321, w319) -> (resulting string=w317:string)  [unwired: 2 in, 1 out]
                n261 = global write "Global 1.vi" "콜라 카메라 값"(w317) -> ()
                n262 = Wait (ms)(milliseconds to wait=u32 300) -> ()  [unwired: 1 out]
              }
              frame #25 {
                n263 = global write "Global 1.vi" "TCP 스위치"(FALSE ("그리퍼 열림")) -> ()
                n264 = Wait Until Next ms Multiple(millisecond multiple=u32 300 ("milliseconds to wait")) -> ()  [unwired: 1 out]
              }
              frame #26 {
                # "콜라 들러가기"
                n265 = global read "Global 1.vi" "콜라 카메라 값"() -> (w357:string)
                n266 = invoke class="PrimaryInterfaceScript" method="Send"(reference=w355, "script"=w357) -> (reference out=w354:refnum<k24>)  [unwired: 2 in, 3 out]
                n267 = Wait (ms)(milliseconds to wait=u32 8000) -> ()  [unwired: 1 out]
              }
              frame #27 {
                n268 = global write "Global 1.vi" "그리퍼 닫힘"(TRUE ("그리퍼 열림")) -> ()
                n269 = Wait (ms)(milliseconds to wait=u32 300) -> ()  [unwired: 1 out]
              }
              frame #28 {
                n270 = global write "Global 1.vi" "그리퍼 닫힘"(FALSE ("그리퍼 열림")) -> ()
                n271 = Wait (ms)(milliseconds to wait=u32 3000) -> ()  [unwired: 1 out]
              }
              frame #29 {
                # "콜라 들어올리기"
                n272 = global read "Global 1.vi" "콜라 드는 자세"() -> (w367:string)
                n273 = invoke class="PrimaryInterfaceScript" method="Send"(reference=w365, "script"=w367) -> (reference out=w364:refnum<k24>)  [unwired: 2 in, 3 out]
                n274 = Wait (ms)(milliseconds to wait=u32 5000) -> ()  [unwired: 1 out]
              }
              frame #30 {
                # "콜라 살짝 빼기"
                n275 = global read "Global 1.vi" "콜라 빼는 자세"() -> (w371:string)
                n276 = invoke class="PrimaryInterfaceScript" method="Send"(reference=w369, "script"=w371) -> (reference out=w368:refnum<k24>)  [unwired: 2 in, 3 out]
                n277 = Wait (ms)(milliseconds to wait=u32 5000) -> ()  [unwired: 1 out]
              }
              frame #31 {
                # "술잔 중간지점으로 이동"
                n278 = global read "Global 1.vi" "술잔 중간지점"() -> (w374:string)
                n279 = invoke class="PrimaryInterfaceScript" method="Send"(reference=w373, "script"=w374) -> (reference out=w372:refnum<k24>)  [unwired: 2 in, 3 out]
                n280 = Wait (ms)(milliseconds to wait=u32 15000) -> ()  [unwired: 1 out]
              }
              frame #32 {
                # "술잔으로 이동"
                n281 = global read "Global 1.vi" "술잔 위로 가는 자세"() -> (w379:string)
                n282 = invoke class="PrimaryInterfaceScript" method="Send"(reference=w377, "script"=w379) -> (reference out=w376:refnum<k24>)  [unwired: 2 in, 3 out]
                n283 = Wait (ms)(milliseconds to wait=u32 5000) -> ()  [unwired: 1 out]
              }
              frame #33 {
                # "미니콜라에 따르기"
                n284 = global read "Global 1.vi" "미니콜라 따르는 자세"() -> (w383:string)
                n285 = invoke class="PrimaryInterfaceScript" method="Send"(reference=w381, "script"=w383) -> (reference out=w380:refnum<k24>)  [unwired: 2 in, 3 out]
                n286 = Wait (ms)(milliseconds to wait=u32 11000) -> ()  [unwired: 1 out]
              }
              frame #34 {
                # "술따르기 중단"
                n287 = global read "Global 1.vi" "술잔 위로 가는 자세"() -> (w387:string)
                n288 = invoke class="PrimaryInterfaceScript" method="Send"(reference=w385, "script"=w387) -> (reference out=w384:refnum<k24>)  [unwired: 2 in, 3 out]
                n289 = Wait (ms)(milliseconds to wait=u32 5000) -> ()  [unwired: 1 out]
              }
              frame #35 {
                # "술잔 중간지점으로 이동"
                n290 = global read "Global 1.vi" "술잔 중간지점"() -> (w390:string)
                n291 = invoke class="PrimaryInterfaceScript" method="Send"(reference=w389, "script"=w390) -> (reference out=w388:refnum<k24>)  [unwired: 2 in, 3 out]
                n292 = Wait (ms)(milliseconds to wait=u32 7000) -> ()  [unwired: 1 out]
              }
              frame #36 {
                # "콜라 뻇던 자세로 복귀"
                n293 = global read "Global 1.vi" "콜라 빼는 자세"() -> (w394:string)
                n294 = invoke class="PrimaryInterfaceScript" method="Send"(reference=w393, "script"=w394) -> (reference out=w392:refnum<k24>)  [unwired: 2 in, 3 out]
                n295 = Wait (ms)(milliseconds to wait=u32 7000) -> ()  [unwired: 1 out]
              }
              frame #37 {
                # "콜라 내려놓으러 가기"
                n296 = global read "Global 1.vi" "콜라 드는 자세"() -> (w399:string)
                n297 = invoke class="PrimaryInterfaceScript" method="Send"(reference=w397, "script"=w399) -> (reference out=w396:refnum<k24>)  [unwired: 2 in, 3 out]
                n298 = Wait (ms)(milliseconds to wait=u32 10000) -> ()  [unwired: 1 out]
              }
              frame #38 {
                # "콜라 내려놓기"
                n299 = global read "Global 1.vi" "콜라로 가는자세"() -> (w403:string)
                n300 = invoke class="PrimaryInterfaceScript" method="Send"(reference=w401, "script"=w403) -> (reference out=w400:refnum<k24>)  [unwired: 2 in, 3 out]
                n301 = Wait (ms)(milliseconds to wait=u32 5000) -> ()  [unwired: 1 out]
              }
              frame #39 {
                # "그리퍼 열기"
                n302 = global write "Global 1.vi" "그리퍼 열림"(TRUE ("그리퍼 열림")) -> ()
                n303 = Wait (ms)(milliseconds to wait=u32 300) -> ()  [unwired: 1 out]
              }
              frame #40 {
                n304 = global write "Global 1.vi" "그리퍼 열림"(FALSE ("그리퍼 열림")) -> ()
                n305 = Wait (ms)(milliseconds to wait=u32 3000) -> ()  [unwired: 1 out]
              }
              frame #41 {
                # "콜라 뻇던 자세로 복귀"
                n306 = global read "Global 1.vi" "콜라 빼는 자세"() -> (w412:string)
                n307 = invoke class="PrimaryInterfaceScript" method="Send"(reference=w411, "script"=w412) -> (reference out=w410:refnum<k24>)  [unwired: 2 in, 3 out]
                n308 = Wait (ms)(milliseconds to wait=u32 5000) -> ()  [unwired: 1 out]
              }
              frame #42 {
                # "초기자세"
                n309 = global read "Global 1.vi" "1자로 서는 자세"() -> (w416:string)
                n310 = invoke class="PrimaryInterfaceScript" method="Send"(reference=w414, "script"=w416) -> ()  [unwired: 2 in, 4 out]
                n311 = Wait (ms)(milliseconds to wait=u32 15000) -> ()  [unwired: 1 out]
              }
              frame #43 {
                n312 = global write "Global 1.vi" "그리퍼 닫힘"(TRUE ("그리퍼 열림")) -> ()
                n313 = Wait (ms)(milliseconds to wait=u32 300) -> ()  [unwired: 1 out]
              }
              frame #44 {
                w419 = ""
                # "그리퍼의 앙다문 일자 입"
                n314 = global write "Global 1.vi" "그리퍼 닫힘"(FALSE ("그리퍼 열림")) -> ()
                n315 = Wait (ms)(milliseconds to wait=u32 3000) -> ()  [unwired: 1 out]
                n316 = global write "Global 1.vi" "잭다니엘 카메라 값"(w419) -> ()
                n317 = global write "Global 1.vi" "콜라 카메라 값"(w419) -> ()
                n318 = global write "Global 1.vi" "토닉 카메라 값"(w419) -> ()
                n319 = global write "Global 1.vi" "짐빔 카메라 값"(w419) -> ()
              }
            }
          }
          frame 2 {
            # "짐빔 : 토닉 = 1: 3"
            # "2nd order"
            n320 = flat-sequence {
              tunnel: w434 -> [w465]
              tunnel: [w464] -> w461
              tunnel: w461 -> [w469]
              tunnel: [w467] -> w460
              tunnel: w460 -> [w472]
              tunnel: [w472] -> w459
              tunnel: w459 -> [w475]
              tunnel: [w475] -> w431
              tunnel: w431 -> [w479]
              tunnel: [w479] -> w430
              tunnel: w430 -> [w486]
              tunnel: [w486] -> w429
              tunnel: w429 -> [w562]
              tunnel: [w562] -> w428
              tunnel: w428 -> [w565]
              tunnel: [w565] -> w427
              tunnel: w427 -> [w569]
              tunnel: [w566] -> w458
              tunnel: w458 -> [w572]
              tunnel: [w572] -> w457
              tunnel: w457 -> [w575]
              tunnel: [w575] -> w456
              tunnel: w456 -> [w577]
              tunnel: [w576] -> w455
              tunnel: w455 -> [w581]
              tunnel: [w580] -> w454
              tunnel: w454 -> [w586]
              tunnel: [w584] -> w453
              tunnel: w453 -> [w589]
              tunnel: [w588] -> w452
              tunnel: w452 -> [w594]
              tunnel: [w592] -> w451
              tunnel: w451 -> [w597]
              tunnel: [w596] -> w450
              tunnel: w450 -> [w602]
              tunnel: [w602] -> w449
              tunnel: w449 -> [w605]
              tunnel: [w605] -> w433
              tunnel: w433 -> [w607]
              tunnel: [w606] -> w432
              tunnel: [w610] -> w426
              tunnel: w432 -> [w611]
              tunnel: w426 -> [w617]
              tunnel: [w617] -> w425
              tunnel: w425 -> [w624]
              tunnel: [w624] -> w424
              tunnel: w424 -> [w700]
              tunnel: [w700] -> w423
              tunnel: w423 -> [w703]
              tunnel: [w703] -> w422
              tunnel: w422 -> [w705]
              tunnel: [w704] -> w448
              tunnel: w448 -> [w710]
              tunnel: [w710] -> w447
              tunnel: w447 -> [w713]
              tunnel: [w713] -> w446
              tunnel: w446 -> [w715]
              tunnel: [w714] -> w445
              tunnel: w445 -> [w719]
              tunnel: [w718] -> w444
              tunnel: w444 -> [w723]
              tunnel: [w722] -> w443
              tunnel: w443 -> [w727]
              tunnel: [w726] -> w442
              tunnel: w442 -> [w731]
              tunnel: [w730] -> w441
              tunnel: w441 -> [w735]
              tunnel: [w734] -> w440
              tunnel: w440 -> [w739]
              tunnel: [w738] -> w439
              tunnel: w439 -> [w743]
              tunnel: [w742] -> w438
              tunnel: [w746] -> w437
              tunnel: w438 -> [w746]
              tunnel: [w749] -> w436
              tunnel: w437 -> [w749]
              tunnel: w436 -> [w753]
              tunnel: [w752] -> w435
              tunnel: w435 -> [w756]
              frame #0 {
                # "초기자세"
                n321 = global read "Global 1.vi" "1자로 서는 자세"() -> (w463:string)
                n322 = invoke class="PrimaryInterfaceScript" method="Send"(reference=w465, "script"=w463) -> (reference out=w464:refnum<k24>)  [unwired: 2 in, 3 out]
                n323 = Wait (ms)(milliseconds to wait=u32 15000) -> ()  [unwired: 1 out]
              }
              frame #1 {
                # "짐빔 보기"
                n324 = global read "Global 1.vi" "짐빔 보는 자세"() -> (w468:string)
                n325 = invoke class="PrimaryInterfaceScript" method="Send"(reference=w469, "script"=w468) -> (reference out=w467:refnum<k24>)  [unwired: 2 in, 3 out]
                n326 = Wait (ms)(milliseconds to wait=u32 15000) -> ()  [unwired: 1 out]
              }
              frame #2 {
                # "그리퍼 열기"
                n327 = global write "Global 1.vi" "그리퍼 열림"(TRUE ("그리퍼 열림")) -> ()
                n328 = Wait (ms)(milliseconds to wait=u32 300) -> ()  [unwired: 1 out]
              }
              frame #3 {
                n329 = global write "Global 1.vi" "그리퍼 열림"(FALSE ("그리퍼 열림")) -> ()
                n330 = Wait (ms)(milliseconds to wait=u32 300) -> ()  [unwired: 1 out]
              }
              frame #4 {
                # "tcp 키는 스위치 보단\n파이썬한테 \n값 보내달라하는\n요청 보내는 걸로 \n바꾸기"
                n331 = global write "Global 1.vi" "몇번 병을 볼것인가"("3" ("몇번 병을 볼것인가")) -> ()
                n332 = global write "Global 1.vi" "TCP 스위치"(TRUE ("그리퍼 열림")) -> ()
                n333 = Wait Until Next ms Multiple(millisecond multiple=u32 500 ("milliseconds to wait")) -> ()  [unwired: 1 out]
              }
              frame #5 {
                n334 = global read "Global 1.vi" "X_부호"() -> (w482:string)
                n335 = global read "Global 1.vi" "Z_부호"() -> (w480:string)
                n336 = global read "Global 1.vi" "Y_부호"() -> (w481:string)
                n337 = case shown="\"1\"" w480 {
                  frame "False", Default {
                  }
                  frame "True" {
                  }
                  frame "2" {
                  }
                  frame "1" {
                    n338 = global read "Global 1.vi" "Z_havetogo"() -> (w488:string)
                    n339 = Decimal String To Number(string=w488) -> (number=w491:i32)  [unwired: 2 in, 1 out]
                    n340 = To Double Precision Float(number=w491) -> (double precision float=w490:dbl)
                    n341 = Format Into String(format string="-%f", w490) -> (resulting string=w487:string)  [unwired: 2 in, 1 out]
                    n342 = global write "Global 1.vi" "Z_havetogo"(w487) -> ()
                  }
                }
                n343 = case shown="\"1\"" w481 {
                  frame "False", Default {
                  }
                  frame "True" {
                  }
                  frame "2" {
                  }
                  frame "1" {
                    n344 = global read "Global 1.vi" "Y_havetogo"() -> (w493:string)
                    n345 = Decimal String To Number(string=w493) -> (number=w496:i32)  [unwired: 2 in, 1 out]
                    n346 = To Double Precision Float(number=w496) -> (double precision float=w494:dbl)
                    n347 = Format Into String(format string="-%f", w494) -> (resulting string=w492:string)  [unwired: 2 in, 1 out]
                    n348 = global write "Global 1.vi" "Y_havetogo"(w492) -> ()
                  }
                }
                n349 = case shown="\"1\"" w482 {
                  frame "False", Default {
                  }
                  frame "True" {
                  }
                  frame "2" {
                  }
                  frame "1" {
                    n350 = global read "Global 1.vi" "X_havetogo"() -> (w498:string)
                    n351 = Decimal String To Number(string=w498) -> (number=w501:i32)  [unwired: 2 in, 1 out]
                    n352 = To Double Precision Float(number=w501) -> (double precision float=w500:dbl)
                    n353 = Format Into String(format string="-%f", w500) -> (resulting string=w497:string)  [unwired: 2 in, 1 out]
                    n354 = global write "Global 1.vi" "X_havetogo"(w497) -> ()
                  }
                }
                n355 = global read "Global 1.vi" "RX_부호"() -> (w485:string)
                n356 = global read "Global 1.vi" "RZ_부호"() -> (w483:string)
                n357 = global read "Global 1.vi" "RY_부호"() -> (w484:string)
                n358 = case shown="\"1\"" w483 {
                  frame "False", Default {
                  }
                  frame "True" {
                  }
                  frame "2" {
                  }
                  frame "1" {
                    n359 = global read "Global 1.vi" "RZ_havetogo"() -> (w503:string)
                    n360 = Decimal String To Number(string=w503) -> (number=w506:i32)  [unwired: 2 in, 1 out]
                    n361 = To Double Precision Float(number=w506) -> (double precision float=w505:dbl)
                    n362 = Format Into String(format string="-%f", w505) -> (resulting string=w502:string)  [unwired: 2 in, 1 out]
                    n363 = global write "Global 1.vi" "RZ_havetogo"(w502) -> ()
                  }
                }
                n364 = case shown="\"1\"" w484 {
                  frame "False", Default {
                  }
                  frame "True" {
                  }
                  frame "2" {
                  }
                  frame "1" {
                    n365 = global read "Global 1.vi" "RY_havetogo"() -> (w508:string)
                    n366 = Decimal String To Number(string=w508) -> (number=w511:i32)  [unwired: 2 in, 1 out]
                    n367 = To Double Precision Float(number=w511) -> (double precision float=w509:dbl)
                    n368 = Format Into String(format string="-%f", w509) -> (resulting string=w507:string)  [unwired: 2 in, 1 out]
                    n369 = global write "Global 1.vi" "RY_havetogo"(w507) -> ()
                  }
                }
                n370 = case shown="\"1\"" w485 {
                  frame "False", Default {
                  }
                  frame "True" {
                  }
                  frame "2" {
                  }
                  frame "1" {
                    n371 = global read "Global 1.vi" "RX_havetogo"() -> (w513:string)
                    n372 = Decimal String To Number(string=w513) -> (number=w516:i32)  [unwired: 2 in, 1 out]
                    n373 = To Double Precision Float(number=w516) -> (double precision float=w515:dbl)
                    n374 = Format Into String(format string="-%f", w515) -> (resulting string=w512:string)  [unwired: 2 in, 1 out]
                    n375 = global write "Global 1.vi" "RX_havetogo"(w512) -> ()
                  }
                }
              }
              frame #6 {
                n376 = global read "Global 1.vi" "X_havetogo"() -> (w528:string)
                n377 = global read "Global 1.vi" "Y_havetogo"() -> (w527:string)
                n378 = global read "Global 1.vi" "Z_havetogo"() -> (w526:string)
                n379 = global read "Global 1.vi" "RX_havetogo"() -> (w525:string)
                n380 = global read "Global 1.vi" "RY_havetogo"() -> (w524:string)
                n381 = global read "Global 1.vi" "RZ_havetogo"() -> (w523:string)
                n382 = Decimal String To Number(string=w526) -> (number=w552:i32)  [unwired: 2 in, 1 out]
                n383 = Decimal String To Number(string=w528) -> (number=w558:i32)  [unwired: 2 in, 1 out]
                n384 = Decimal String To Number(string=w527) -> (number=w555:i32)  [unwired: 2 in, 1 out]
                n385 = Decimal String To Number(string=w525) -> (number=w549:i32)  [unwired: 2 in, 1 out]
                n386 = Decimal String To Number(string=w524) -> (number=w546:i32)  [unwired: 2 in, 1 out]
                n387 = Decimal String To Number(string=w523) -> (number=w543:i32)  [unwired: 2 in, 1 out]
                n388 = To Double Precision Float(number=w552) -> (double precision float=w554:dbl)
                n389 = To Double Precision Float(number=w558) -> (double precision float=w560:dbl)
                n390 = To Double Precision Float(number=w555) -> (double precision float=w557:dbl)
                n391 = To Double Precision Float(number=w549) -> (double precision float=w551:dbl)
                n392 = To Double Precision Float(number=w546) -> (double precision float=w548:dbl)
                n393 = Multiply(x=w560, y=0.001) -> (x*y=w542:dbl)
                n394 = Multiply(x=w554, y=0.001) -> (x*y=w538:dbl)
                n395 = Multiply(x=w557, y=0.001) -> (x*y=w540:dbl)
                n396 = Multiply(x=w551, y=0.001) -> (x*y=w536:dbl)
                n397 = global read "Global 1.vi" "x"() -> (w522:dbl)
                n398 = Multiply(x=w548, y=0.001) -> (x*y=w534:dbl)
                n399 = global read "Global 1.vi" "y"() -> (w521:dbl)
                n400 = global read "Global 1.vi" "rx"() -> (w519:dbl)
                n401 = global read "Global 1.vi" "z"() -> (w520:dbl)
                n402 = To Double Precision Float(number=w543) -> (double precision float=w545:dbl)
                n403 = Add(x=w522, y=w542) -> (x+y=w541:dbl)
                n404 = Multiply(x=w545, y=0.001) -> (x*y=w532:dbl)
                n405 = Add(x=w538, y=w520) -> (x+y=w537:dbl)
                n406 = Add(x=w540, y=w521) -> (x+y=w539:dbl)
                n407 = global read "Global 1.vi" "ry"() -> (w517:dbl)
                n408 = global read "Global 1.vi" "rz"() -> (w518:dbl)
                n409 = Add(x=w536, y=w519) -> (x+y=w535:dbl)
                n410 = Add(x=w534, y=w517) -> (x+y=w533:dbl)
                n411 = Add(x=w532, y=w518) -> (x+y=w531:dbl)
                n412 = Format Into String(format string="movej( get_inverse_kin(p[%f, %f, %f, %f, %f, %f]), a= 0.5, v=0.25, t=0, r=0)", w541, w539, w537, w535, w533, w531) -> (resulting string=w529:string)  [unwired: 2 in, 1 out]
                n413 = global write "Global 1.vi" "짐빔 카메라 값"(w529) -> ()
                n414 = Wait (ms)(milliseconds to wait=u32 300) -> ()  [unwired: 1 out]
              }
              frame #7 {
                n415 = global write "Global 1.vi" "TCP 스위치"(FALSE ("그리퍼 열림")) -> ()
                n416 = Wait Until Next ms Multiple(millisecond multiple=u32 300 ("milliseconds to wait")) -> ()  [unwired: 1 out]
              }
              frame #8 {
                # "짐빔 위치로 가기"
                n417 = global read "Global 1.vi" "짐빔 카메라 값"() -> (w568:string)
                n418 = invoke class="PrimaryInterfaceScript" method="Send"(reference=w569, "script"=w568) -> (reference out=w566:refnum<k24>)  [unwired: 2 in, 3 out]
                n419 = Wait (ms)(milliseconds to wait=u32 7000) -> ()  [unwired: 1 out]
              }
              frame #9 {
                # "그리퍼 닫기"
                n420 = global write "Global 1.vi" "그리퍼 닫힘"(TRUE ("그리퍼 열림")) -> ()
                n421 = Wait (ms)(milliseconds to wait=u32 300) -> ()  [unwired: 1 out]
              }
              frame #10 {
                n422 = global write "Global 1.vi" "그리퍼 닫힘"(FALSE ("그리퍼 열림")) -> ()
                n423 = Wait (ms)(milliseconds to wait=u32 3000) -> ()  [unwired: 1 out]
              }
              frame #11 {
                # "짐빔 들기"
                n424 = global read "Global 1.vi" "짐빔 들어올리는 자세"() -> (w579:string)
                n425 = invoke class="PrimaryInterfaceScript" method="Send"(reference=w577, "script"=w579) -> (reference out=w576:refnum<k24>)  [unwired: 2 in, 3 out]
                n426 = Wait (ms)(milliseconds to wait=u32 5000) -> ()  [unwired: 1 out]
              }
              frame #12 {
                # "술잔 쪽으로 이동"
                n427 = global read "Global 1.vi" "술잔 위로 가는 자세 2"() -> (w582:string)
                n428 = invoke class="PrimaryInterfaceScript" method="Send"(reference=w581, "script"=w582) -> (reference out=w580:refnum<k24>)  [unwired: 2 in, 3 out]
                n429 = Wait (ms)(milliseconds to wait=u32 15000) -> ()  [unwired: 1 out]
              }
              frame #13 {
                # "술따르기"
                n430 = global read "Global 1.vi" "술 따르는 자세 2"() -> (w585:string)
                n431 = invoke class="PrimaryInterfaceScript" method="Send"(reference=w586, "script"=w585) -> (reference out=w584:refnum<k24>)  [unwired: 2 in, 3 out]
                n432 = Wait (ms)(milliseconds to wait=u32 9000) -> ()  [unwired: 1 out]
              }
              frame #14 {
                # "술따르기 중단"
                n433 = global read "Global 1.vi" "술잔 위로 가는 자세 2"() -> (w590:string)
                n434 = invoke class="PrimaryInterfaceScript" method="Send"(reference=w589, "script"=w590) -> (reference out=w588:refnum<k24>)  [unwired: 2 in, 3 out]
                n435 = Wait (ms)(milliseconds to wait=u32 4000) -> ()  [unwired: 1 out]
              }
              frame #15 {
                # "짐빔 들었던 곳으로"
                n436 = global read "Global 1.vi" "짐빔 들어올리는 자세"() -> (w593:string)
                n437 = invoke class="PrimaryInterfaceScript" method="Send"(reference=w594, "script"=w593) -> (reference out=w592:refnum<k24>)  [unwired: 2 in, 3 out]
                n438 = Wait (ms)(milliseconds to wait=u32 10000) -> ()  [unwired: 1 out]
              }
              frame #16 {
                # "짐빔 내려놓기"
                n439 = global read "Global 1.vi" "짐빔 위치로 가는 자세"() -> (w599:string)
                n440 = invoke class="PrimaryInterfaceScript" method="Send"(reference=w597, "script"=w599) -> (reference out=w596:refnum<k24>)  [unwired: 2 in, 3 out]
                n441 = Wait (ms)(milliseconds to wait=u32 5000) -> ()  [unwired: 1 out]
              }
              frame #17 {
                # "그리퍼 열기"
                n442 = global write "Global 1.vi" "그리퍼 열림"(TRUE ("그리퍼 열림")) -> ()
                n443 = Wait (ms)(milliseconds to wait=u32 300) -> ()  [unwired: 1 out]
              }
              frame #18 {
                n444 = global write "Global 1.vi" "그리퍼 열림"(FALSE ("그리퍼 열림")) -> ()
                n445 = Wait (ms)(milliseconds to wait=u32 3000) -> ()  [unwired: 1 out]
              }
              frame #19 {
                # "짐빔에서 토닉으로 이동준비"
                n446 = global read "Global 1.vi" "짐빔 토닉 이동 준비자세"() -> (w609:string)
                n447 = invoke class="PrimaryInterfaceScript" method="Send"(reference=w607, "script"=w609) -> (reference out=w606:refnum<k24>)  [unwired: 2 in, 3 out]
                n448 = Wait (ms)(milliseconds to wait=u32 5000) -> ()  [unwired: 1 out]
              }
              frame #20 {
                # "토닉보러가기"
                n449 = global read "Global 1.vi" "토닉 보는 자세"() -> (w613:string)
                n450 = invoke class="PrimaryInterfaceScript" method="Send"(reference=w611, "script"=w613) -> (reference out=w610:refnum<k24>)  [unwired: 2 in, 3 out]
                n451 = Wait (ms)(milliseconds to wait=u32 8000) -> ()  [unwired: 1 out]
              }
              frame #21 {
                # "tcp 키는 스위치 보단\n파이썬한테 \n값 보내달라하는\n요청 보내는 걸로 \n바꾸기"
                n452 = global write "Global 1.vi" "몇번 병을 볼것인가"("4" ("몇번 병을 볼것인가")) -> ()
                n453 = global write "Global 1.vi" "TCP 스위치"(TRUE ("그리퍼 열림")) -> ()
                n454 = Wait Until Next ms Multiple(millisecond multiple=u32 500 ("milliseconds to wait")) -> ()  [unwired: 1 out]
              }
              frame #22 {
                n455 = global read "Global 1.vi" "X_부호"() -> (w620:string)
                n456 = global read "Global 1.vi" "Z_부호"() -> (w618:string)
                n457 = global read "Global 1.vi" "Y_부호"() -> (w619:string)
                n458 = case shown="\"1\"" w618 {
                  frame "False", Default {
                  }
                  frame "True" {
                  }
                  frame "2" {
                  }
                  frame "1" {
                    n459 = global read "Global 1.vi" "Z_havetogo"() -> (w626:string)
                    n460 = Decimal String To Number(string=w626) -> (number=w629:i32)  [unwired: 2 in, 1 out]
                    n461 = To Double Precision Float(number=w629) -> (double precision float=w628:dbl)
                    n462 = Format Into String(format string="-%f", w628) -> (resulting string=w625:string)  [unwired: 2 in, 1 out]
                    n463 = global write "Global 1.vi" "Z_havetogo"(w625) -> ()
                  }
                }
                n464 = case shown="\"1\"" w619 {
                  frame "False", Default {
                  }
                  frame "True" {
                  }
                  frame "2" {
                  }
                  frame "1" {
                    n465 = global read "Global 1.vi" "Y_havetogo"() -> (w631:string)
                    n466 = Decimal String To Number(string=w631) -> (number=w634:i32)  [unwired: 2 in, 1 out]
                    n467 = To Double Precision Float(number=w634) -> (double precision float=w632:dbl)
                    n468 = Format Into String(format string="-%f", w632) -> (resulting string=w630:string)  [unwired: 2 in, 1 out]
                    n469 = global write "Global 1.vi" "Y_havetogo"(w630) -> ()
                  }
                }
                n470 = case shown="\"1\"" w620 {
                  frame "False", Default {
                  }
                  frame "True" {
                  }
                  frame "2" {
                  }
                  frame "1" {
                    n471 = global read "Global 1.vi" "X_havetogo"() -> (w636:string)
                    n472 = Decimal String To Number(string=w636) -> (number=w639:i32)  [unwired: 2 in, 1 out]
                    n473 = To Double Precision Float(number=w639) -> (double precision float=w638:dbl)
                    n474 = Format Into String(format string="-%f", w638) -> (resulting string=w635:string)  [unwired: 2 in, 1 out]
                    n475 = global write "Global 1.vi" "X_havetogo"(w635) -> ()
                  }
                }
                n476 = global read "Global 1.vi" "RX_부호"() -> (w623:string)
                n477 = global read "Global 1.vi" "RZ_부호"() -> (w621:string)
                n478 = global read "Global 1.vi" "RY_부호"() -> (w622:string)
                n479 = case shown="\"1\"" w621 {
                  frame "False", Default {
                  }
                  frame "True" {
                  }
                  frame "2" {
                  }
                  frame "1" {
                    n480 = global read "Global 1.vi" "RZ_havetogo"() -> (w641:string)
                    n481 = Decimal String To Number(string=w641) -> (number=w644:i32)  [unwired: 2 in, 1 out]
                    n482 = To Double Precision Float(number=w644) -> (double precision float=w643:dbl)
                    n483 = Format Into String(format string="-%f", w643) -> (resulting string=w640:string)  [unwired: 2 in, 1 out]
                    n484 = global write "Global 1.vi" "RZ_havetogo"(w640) -> ()
                  }
                }
                n485 = case shown="\"1\"" w622 {
                  frame "False", Default {
                  }
                  frame "True" {
                  }
                  frame "2" {
                  }
                  frame "1" {
                    n486 = global read "Global 1.vi" "RY_havetogo"() -> (w646:string)
                    n487 = Decimal String To Number(string=w646) -> (number=w649:i32)  [unwired: 2 in, 1 out]
                    n488 = To Double Precision Float(number=w649) -> (double precision float=w647:dbl)
                    n489 = Format Into String(format string="-%f", w647) -> (resulting string=w645:string)  [unwired: 2 in, 1 out]
                    n490 = global write "Global 1.vi" "RY_havetogo"(w645) -> ()
                  }
                }
                n491 = case shown="\"1\"" w623 {
                  frame "False", Default {
                  }
                  frame "True" {
                  }
                  frame "2" {
                  }
                  frame "1" {
                    n492 = global read "Global 1.vi" "RX_havetogo"() -> (w651:string)
                    n493 = Decimal String To Number(string=w651) -> (number=w654:i32)  [unwired: 2 in, 1 out]
                    n494 = To Double Precision Float(number=w654) -> (double precision float=w653:dbl)
                    n495 = Format Into String(format string="-%f", w653) -> (resulting string=w650:string)  [unwired: 2 in, 1 out]
                    n496 = global write "Global 1.vi" "RX_havetogo"(w650) -> ()
                  }
                }
              }
              frame #23 {
                n497 = global read "Global 1.vi" "X_havetogo"() -> (w666:string)
                n498 = global read "Global 1.vi" "Y_havetogo"() -> (w665:string)
                n499 = global read "Global 1.vi" "Z_havetogo"() -> (w664:string)
                n500 = global read "Global 1.vi" "RX_havetogo"() -> (w663:string)
                n501 = global read "Global 1.vi" "RY_havetogo"() -> (w662:string)
                n502 = global read "Global 1.vi" "RZ_havetogo"() -> (w661:string)
                n503 = Decimal String To Number(string=w664) -> (number=w690:i32)  [unwired: 2 in, 1 out]
                n504 = Decimal String To Number(string=w666) -> (number=w696:i32)  [unwired: 2 in, 1 out]
                n505 = Decimal String To Number(string=w665) -> (number=w693:i32)  [unwired: 2 in, 1 out]
                n506 = Decimal String To Number(string=w663) -> (number=w687:i32)  [unwired: 2 in, 1 out]
                n507 = Decimal String To Number(string=w662) -> (number=w684:i32)  [unwired: 2 in, 1 out]
                n508 = Decimal String To Number(string=w661) -> (number=w681:i32)  [unwired: 2 in, 1 out]
                n509 = To Double Precision Float(number=w690) -> (double precision float=w692:dbl)
                n510 = To Double Precision Float(number=w696) -> (double precision float=w698:dbl)
                n511 = To Double Precision Float(number=w693) -> (double precision float=w695:dbl)
                n512 = To Double Precision Float(number=w687) -> (double precision float=w689:dbl)
                n513 = To Double Precision Float(number=w684) -> (double precision float=w686:dbl)
                n514 = Multiply(x=w698, y=0.001) -> (x*y=w680:dbl)
                n515 = Multiply(x=w692, y=0.001) -> (x*y=w676:dbl)
                n516 = Multiply(x=w695, y=0.001) -> (x*y=w678:dbl)
                n517 = Multiply(x=w689, y=0.001) -> (x*y=w674:dbl)
                n518 = global read "Global 1.vi" "x"() -> (w660:dbl)
                n519 = Multiply(x=w686, y=0.001) -> (x*y=w672:dbl)
                n520 = global read "Global 1.vi" "y"() -> (w659:dbl)
                n521 = global read "Global 1.vi" "rx"() -> (w657:dbl)
                n522 = global read "Global 1.vi" "z"() -> (w658:dbl)
                n523 = To Double Precision Float(number=w681) -> (double precision float=w683:dbl)
                n524 = Add(x=w660, y=w680) -> (x+y=w679:dbl)
                n525 = Multiply(x=w683, y=0.001) -> (x*y=w670:dbl)
                n526 = Add(x=w676, y=w658) -> (x+y=w675:dbl)
                n527 = Add(x=w678, y=w659) -> (x+y=w677:dbl)
                n528 = global read "Global 1.vi" "ry"() -> (w655:dbl)
                n529 = global read "Global 1.vi" "rz"() -> (w656:dbl)
                n530 = Add(x=w674, y=w657) -> (x+y=w673:dbl)
                n531 = Add(x=w672, y=w655) -> (x+y=w671:dbl)
                n532 = Add(x=w670, y=w656) -> (x+y=w669:dbl)
                n533 = Format Into String(format string="movej( get_inverse_kin(p[%f, %f, %f, %f, %f, %f]), a= 0.5, v=0.25, t=0, r=0)", w679, w677, w675, w673, w671, w669) -> (resulting string=w667:string)  [unwired: 2 in, 1 out]
                n534 = global write "Global 1.vi" "토닉 카메라 값"(w667) -> ()
                n535 = Wait (ms)(milliseconds to wait=u32 300) -> ()  [unwired: 1 out]
              }
              frame #24 {
                n536 = global write "Global 1.vi" "TCP 스위치"(FALSE ("그리퍼 열림")) -> ()
                n537 = Wait Until Next ms Multiple(millisecond multiple=u32 300 ("milliseconds to wait")) -> ()  [unwired: 1 out]
              }
              frame #25 {
                # "토닉 들러가기"
                n538 = global read "Global 1.vi" "토닉 카메라 값"() -> (w707:string)
                n539 = invoke class="PrimaryInterfaceScript" method="Send"(reference=w705, "script"=w707) -> (reference out=w704:refnum<k24>)  [unwired: 2 in, 3 out]
                n540 = Wait (ms)(milliseconds to wait=u32 8000) -> ()  [unwired: 1 out]
              }
              frame #26 {
                n541 = global write "Global 1.vi" "그리퍼 닫힘"(TRUE ("그리퍼 열림")) -> ()
                n542 = Wait (ms)(milliseconds to wait=u32 300) -> ()  [unwired: 1 out]
              }
              frame #27 {
                n543 = global write "Global 1.vi" "그리퍼 닫힘"(FALSE ("그리퍼 열림")) -> ()
                n544 = Wait (ms)(milliseconds to wait=u32 3000) -> ()  [unwired: 1 out]
              }
              frame #28 {
                # "토닉 들어올리기"
                n545 = global read "Global 1.vi" "토닉 드는 자세"() -> (w717:string)
                n546 = invoke class="PrimaryInterfaceScript" method="Send"(reference=w715, "script"=w717) -> (reference out=w714:refnum<k24>)  [unwired: 2 in, 3 out]
                n547 = Wait (ms)(milliseconds to wait=u32 5000) -> ()  [unwired: 1 out]
              }
              frame #29 {
                # "토닉 살짝 빼기"
                n548 = global read "Global 1.vi" "토닉 빼는 자세"() -> (w721:string)
                n549 = invoke class="PrimaryInterfaceScript" method="Send"(reference=w719, "script"=w721) -> (reference out=w718:refnum<k24>)  [unwired: 2 in, 3 out]
                n550 = Wait (ms)(milliseconds to wait=u32 7000) -> ()  [unwired: 1 out]
              }
              frame #30 {
                # "술잔으로 이동"
                n551 = global read "Global 1.vi" "술잔 위로 가는 자세 2"() -> (w725:string)
                n552 = invoke class="PrimaryInterfaceScript" method="Send"(reference=w723, "script"=w725) -> (reference out=w722:refnum<k24>)  [unwired: 2 in, 3 out]
                n553 = Wait (ms)(milliseconds to wait=u32 12000) -> ()  [unwired: 1 out]
              }
              frame #31 {
                # "술잔에 따르기"
                n554 = global read "Global 1.vi" "술 따르는 자세 2"() -> (w729:string)
                n555 = invoke class="PrimaryInterfaceScript" method="Send"(reference=w727, "script"=w729) -> (reference out=w726:refnum<k24>)  [unwired: 2 in, 3 out]
                n556 = Wait (ms)(milliseconds to wait=u32 13000) -> ()  [unwired: 1 out]
              }
              frame #32 {
                # "술따르기 중단"
                n557 = global read "Global 1.vi" "술잔 위로 가는 자세 2"() -> (w733:string)
                n558 = invoke class="PrimaryInterfaceScript" method="Send"(reference=w731, "script"=w733) -> (reference out=w730:refnum<k24>)  [unwired: 2 in, 3 out]
                n559 = Wait (ms)(milliseconds to wait=u32 5000) -> ()  [unwired: 1 out]
              }
              frame #33 {
                # "토닉 뻇던 자세로 복귀"
                n560 = global read "Global 1.vi" "토닉 빼는 자세"() -> (w736:string)
                n561 = invoke class="PrimaryInterfaceScript" method="Send"(reference=w735, "script"=w736) -> (reference out=w734:refnum<k24>)  [unwired: 2 in, 3 out]
                n562 = Wait (ms)(milliseconds to wait=u32 9000) -> ()  [unwired: 1 out]
              }
              frame #34 {
                # "토닉 내려놓으러 가기"
                n563 = global read "Global 1.vi" "토닉 드는 자세"() -> (w741:string)
                n564 = invoke class="PrimaryInterfaceScript" method="Send"(reference=w739, "script"=w741) -> (reference out=w738:refnum<k24>)  [unwired: 2 in, 3 out]
                n565 = Wait (ms)(milliseconds to wait=u32 7000) -> ()  [unwired: 1 out]
              }
              frame #35 {
                # "토닉 내려놓기"
                n566 = global read "Global 1.vi" "토닉 가는자세"() -> (w745:string)
                n567 = invoke class="PrimaryInterfaceScript" method="Send"(reference=w743, "script"=w745) -> (reference out=w742:refnum<k24>)  [unwired: 2 in, 3 out]
                n568 = Wait (ms)(milliseconds to wait=u32 5000) -> ()  [unwired: 1 out]
              }
              frame #36 {
                # "그리퍼 열기"
                n569 = global write "Global 1.vi" "그리퍼 열림"(TRUE ("그리퍼 열림")) -> ()
                n570 = Wait (ms)(milliseconds to wait=u32 300) -> ()  [unwired: 1 out]
              }
              frame #37 {
                n571 = global write "Global 1.vi" "그리퍼 열림"(FALSE ("그리퍼 열림")) -> ()
                n572 = Wait (ms)(milliseconds to wait=u32 3000) -> ()  [unwired: 1 out]
              }
              frame #38 {
                # "토닉 뻇던 자세로 복귀"
                n573 = global read "Global 1.vi" "토닉 빼는 자세"() -> (w754:string)
                n574 = invoke class="PrimaryInterfaceScript" method="Send"(reference=w753, "script"=w754) -> (reference out=w752:refnum<k24>)  [unwired: 2 in, 3 out]
                n575 = Wait (ms)(milliseconds to wait=u32 5000) -> ()  [unwired: 1 out]
              }
              frame #39 {
                # "초기자세"
                n576 = global read "Global 1.vi" "1자로 서는 자세"() -> (w758:string)
                n577 = invoke class="PrimaryInterfaceScript" method="Send"(reference=w756, "script"=w758) -> ()  [unwired: 2 in, 4 out]
                n578 = Wait (ms)(milliseconds to wait=u32 15000) -> ()  [unwired: 1 out]
              }
              frame #40 {
                n579 = global write "Global 1.vi" "그리퍼 닫힘"(TRUE ("그리퍼 열림")) -> ()
                n580 = Wait (ms)(milliseconds to wait=u32 300) -> ()  [unwired: 1 out]
              }
              frame #41 {
                w761 = ""
                # "그리퍼의 앙다문 일자 입"
                n581 = global write "Global 1.vi" "그리퍼 닫힘"(FALSE ("그리퍼 열림")) -> ()
                n582 = Wait (ms)(milliseconds to wait=u32 3000) -> ()  [unwired: 1 out]
                n583 = global write "Global 1.vi" "잭다니엘 카메라 값"(w761) -> ()
                n584 = global write "Global 1.vi" "콜라 카메라 값"(w761) -> ()
                n585 = global write "Global 1.vi" "토닉 카메라 값"(w761) -> ()
                n586 = global write "Global 1.vi" "짐빔 카메라 값"(w761) -> ()
              }
            }
          }
          frame 3 {
            # "multi order"
          }
          frame 4 {
            # "짐빔 : 우유 = 1 : 3"
            # "3rd order"
            n587 = flat-sequence {
              tunnel: w764 -> [w807]
              tunnel: [w806] -> w803
              tunnel: w803 -> [w811]
              tunnel: [w809] -> w802
              tunnel: w802 -> [w814]
              tunnel: [w814] -> w801
              tunnel: w801 -> [w817]
              tunnel: [w817] -> w800
              tunnel: w800 -> [w821]
              tunnel: [w821] -> w799
              tunnel: w799 -> [w828]
              tunnel: [w828] -> w798
              tunnel: w798 -> [w904]
              tunnel: [w904] -> w797
              tunnel: w797 -> [w907]
              tunnel: [w907] -> w796
              tunnel: w796 -> [w911]
              tunnel: [w908] -> w795
              tunnel: w795 -> [w914]
              tunnel: [w914] -> w794
              tunnel: w794 -> [w917]
              tunnel: [w917] -> w793
              tunnel: w793 -> [w919]
              tunnel: [w918] -> w792
              tunnel: w792 -> [w923]
              tunnel: [w922] -> w791
              tunnel: w791 -> [w928]
              tunnel: [w926] -> w790
              tunnel: w790 -> [w931]
              tunnel: [w930] -> w789
              tunnel: w789 -> [w936]
              tunnel: [w934] -> w788
              tunnel: w788 -> [w939]
              tunnel: [w938] -> w787
              tunnel: w787 -> [w944]
              tunnel: [w944] -> w786
              tunnel: w786 -> [w947]
              tunnel: [w947] -> w785
              tunnel: w785 -> [w949]
              tunnel: [w948] -> w784
              tunnel: [w952] -> w783
              tunnel: w784 -> [w953]
              tunnel: w783 -> [w959]
              tunnel: [w959] -> w782
              tunnel: w782 -> [w966]
              tunnel: [w966] -> w781
              tunnel: w781 -> [w1042]
              tunnel: [w1042] -> w780
              tunnel: w780 -> [w1045]
              tunnel: [w1045] -> w779
              tunnel: w779 -> [w1047]
              tunnel: [w1046] -> w778
              tunnel: w778 -> [w1052]
              tunnel: [w1052] -> w777
              tunnel: w777 -> [w1055]
              tunnel: [w1055] -> w776
              tunnel: w776 -> [w1057]
              tunnel: [w1056] -> w775
              tunnel: w775 -> [w1061]
              tunnel: [w1060] -> w774
              tunnel: w774 -> [w1065]
              tunnel: [w1064] -> w773
              tunnel: w773 -> [w1069]
              tunnel: [w1068] -> w772
              tunnel: w772 -> [w1073]
              tunnel: [w1072] -> w771
              tunnel: w771 -> [w1077]
              tunnel: [w1076] -> w770
              tunnel: w770 -> [w1081]
              tunnel: [w1080] -> w769
              tunnel: w769 -> [w1085]
              tunnel: [w1084] -> w768
              tunnel: [w1088] -> w767
              tunnel: w768 -> [w1088]
              tunnel: [w1091] -> w766
              tunnel: w767 -> [w1091]
              tunnel: w766 -> [w1095]
              tunnel: [w1094] -> w765
              tunnel: w765 -> [w1098]
              frame #0 {
                # "초기자세"
                n588 = global read "Global 1.vi" "1자로 서는 자세"() -> (w805:string)
                n589 = invoke class="PrimaryInterfaceScript" method="Send"(reference=w807, "script"=w805) -> (reference out=w806:refnum<k24>)  [unwired: 2 in, 3 out]
                n590 = Wait (ms)(milliseconds to wait=u32 15000) -> ()  [unwired: 1 out]
              }
              frame #1 {
                # "짐빔 보기"
                n591 = global read "Global 1.vi" "짐빔 보는 자세"() -> (w810:string)
                n592 = invoke class="PrimaryInterfaceScript" method="Send"(reference=w811, "script"=w810) -> (reference out=w809:refnum<k24>)  [unwired: 2 in, 3 out]
                n593 = Wait (ms)(milliseconds to wait=u32 15000) -> ()  [unwired: 1 out]
              }
              frame #2 {
                # "그리퍼 열기"
                n594 = global write "Global 1.vi" "그리퍼 열림"(TRUE ("그리퍼 열림")) -> ()
                n595 = Wait (ms)(milliseconds to wait=u32 300) -> ()  [unwired: 1 out]
              }
              frame #3 {
                n596 = global write "Global 1.vi" "그리퍼 열림"(FALSE ("그리퍼 열림")) -> ()
                n597 = Wait (ms)(milliseconds to wait=u32 300) -> ()  [unwired: 1 out]
              }
              frame #4 {
                # "tcp 키는 스위치 보단\n파이썬한테 \n값 보내달라하는\n요청 보내는 걸로 \n바꾸기"
                n598 = global write "Global 1.vi" "몇번 병을 볼것인가"("3" ("몇번 병을 볼것인가")) -> ()
                n599 = global write "Global 1.vi" "TCP 스위치"(TRUE ("그리퍼 열림")) -> ()
                n600 = Wait (ms)(milliseconds to wait=u32 200) -> ()  [unwired: 1 out]
              }
              frame #5 {
                n601 = global read "Global 1.vi" "X_부호"() -> (w824:string)
                n602 = global read "Global 1.vi" "Z_부호"() -> (w822:string)
                n603 = global read "Global 1.vi" "Y_부호"() -> (w823:string)
                n604 = case shown="\"1\"" w822 {
                  frame "False", Default {
                  }
                  frame "True" {
                  }
                  frame "2" {
                  }
                  frame "1" {
                    n605 = global read "Global 1.vi" "Z_havetogo"() -> (w830:string)
                    n606 = Decimal String To Number(string=w830) -> (number=w833:i32)  [unwired: 2 in, 1 out]
                    n607 = To Double Precision Float(number=w833) -> (double precision float=w832:dbl)
                    n608 = Format Into String(format string="-%f", w832) -> (resulting string=w829:string)  [unwired: 2 in, 1 out]
                    n609 = global write "Global 1.vi" "Z_havetogo"(w829) -> ()
                  }
                }
                n610 = case shown="\"1\"" w823 {
                  frame "False", Default {
                  }
                  frame "True" {
                  }
                  frame "2" {
                  }
                  frame "1" {
                    n611 = global read "Global 1.vi" "Y_havetogo"() -> (w835:string)
                    n612 = Decimal String To Number(string=w835) -> (number=w838:i32)  [unwired: 2 in, 1 out]
                    n613 = To Double Precision Float(number=w838) -> (double precision float=w836:dbl)
                    n614 = Format Into String(format string="-%f", w836) -> (resulting string=w834:string)  [unwired: 2 in, 1 out]
                    n615 = global write "Global 1.vi" "Y_havetogo"(w834) -> ()
                  }
                }
                n616 = case shown="\"1\"" w824 {
                  frame "False", Default {
                  }
                  frame "True" {
                  }
                  frame "2" {
                  }
                  frame "1" {
                    n617 = global read "Global 1.vi" "X_havetogo"() -> (w840:string)
                    n618 = Decimal String To Number(string=w840) -> (number=w843:i32)  [unwired: 2 in, 1 out]
                    n619 = To Double Precision Float(number=w843) -> (double precision float=w842:dbl)
                    n620 = Format Into String(format string="-%f", w842) -> (resulting string=w839:string)  [unwired: 2 in, 1 out]
                    n621 = global write "Global 1.vi" "X_havetogo"(w839) -> ()
                  }
                }
                n622 = global read "Global 1.vi" "RX_부호"() -> (w827:string)
                n623 = global read "Global 1.vi" "RZ_부호"() -> (w825:string)
                n624 = global read "Global 1.vi" "RY_부호"() -> (w826:string)
                n625 = case shown="\"1\"" w825 {
                  frame "False", Default {
                  }
                  frame "True" {
                  }
                  frame "2" {
                  }
                  frame "1" {
                    n626 = global read "Global 1.vi" "RZ_havetogo"() -> (w845:string)
                    n627 = Decimal String To Number(string=w845) -> (number=w848:i32)  [unwired: 2 in, 1 out]
                    n628 = To Double Precision Float(number=w848) -> (double precision float=w847:dbl)
                    n629 = Format Into String(format string="-%f", w847) -> (resulting string=w844:string)  [unwired: 2 in, 1 out]
                    n630 = global write "Global 1.vi" "RZ_havetogo"(w844) -> ()
                  }
                }
                n631 = case shown="\"1\"" w826 {
                  frame "False", Default {
                  }
                  frame "True" {
                  }
                  frame "2" {
                  }
                  frame "1" {
                    n632 = global read "Global 1.vi" "RY_havetogo"() -> (w850:string)
                    n633 = Decimal String To Number(string=w850) -> (number=w853:i32)  [unwired: 2 in, 1 out]
                    n634 = To Double Precision Float(number=w853) -> (double precision float=w851:dbl)
                    n635 = Format Into String(format string="-%f", w851) -> (resulting string=w849:string)  [unwired: 2 in, 1 out]
                    n636 = global write "Global 1.vi" "RY_havetogo"(w849) -> ()
                  }
                }
                n637 = case shown="\"1\"" w827 {
                  frame "False", Default {
                  }
                  frame "True" {
                  }
                  frame "2" {
                  }
                  frame "1" {
                    n638 = global read "Global 1.vi" "RX_havetogo"() -> (w855:string)
                    n639 = Decimal String To Number(string=w855) -> (number=w858:i32)  [unwired: 2 in, 1 out]
                    n640 = To Double Precision Float(number=w858) -> (double precision float=w857:dbl)
                    n641 = Format Into String(format string="-%f", w857) -> (resulting string=w854:string)  [unwired: 2 in, 1 out]
                    n642 = global write "Global 1.vi" "RX_havetogo"(w854) -> ()
                  }
                }
              }
              frame #6 {
                n643 = global read "Global 1.vi" "X_havetogo"() -> (w870:string)
                n644 = global read "Global 1.vi" "Y_havetogo"() -> (w869:string)
                n645 = global read "Global 1.vi" "Z_havetogo"() -> (w868:string)
                n646 = global read "Global 1.vi" "RX_havetogo"() -> (w867:string)
                n647 = global read "Global 1.vi" "RY_havetogo"() -> (w866:string)
                n648 = global read "Global 1.vi" "RZ_havetogo"() -> (w865:string)
                n649 = Decimal String To Number(string=w868) -> (number=w894:i32)  [unwired: 2 in, 1 out]
                n650 = Decimal String To Number(string=w870) -> (number=w900:i32)  [unwired: 2 in, 1 out]
                n651 = Decimal String To Number(string=w869) -> (number=w897:i32)  [unwired: 2 in, 1 out]
                n652 = Decimal String To Number(string=w867) -> (number=w891:i32)  [unwired: 2 in, 1 out]
                n653 = Decimal String To Number(string=w866) -> (number=w888:i32)  [unwired: 2 in, 1 out]
                n654 = Decimal String To Number(string=w865) -> (number=w885:i32)  [unwired: 2 in, 1 out]
                n655 = To Double Precision Float(number=w894) -> (double precision float=w896:dbl)
                n656 = To Double Precision Float(number=w900) -> (double precision float=w902:dbl)
                n657 = To Double Precision Float(number=w897) -> (double precision float=w899:dbl)
                n658 = To Double Precision Float(number=w891) -> (double precision float=w893:dbl)
                n659 = To Double Precision Float(number=w888) -> (double precision float=w890:dbl)
                n660 = Multiply(x=w902, y=0.001) -> (x*y=w884:dbl)
                n661 = Multiply(x=w896, y=0.001) -> (x*y=w880:dbl)
                n662 = Multiply(x=w899, y=0.001) -> (x*y=w882:dbl)
                n663 = Multiply(x=w893, y=0.001) -> (x*y=w878:dbl)
                n664 = global read "Global 1.vi" "x"() -> (w864:dbl)
                n665 = Multiply(x=w890, y=0.001) -> (x*y=w876:dbl)
                n666 = global read "Global 1.vi" "y"() -> (w863:dbl)
                n667 = global read "Global 1.vi" "rx"() -> (w861:dbl)
                n668 = global read "Global 1.vi" "z"() -> (w862:dbl)
                n669 = To Double Precision Float(number=w885) -> (double precision float=w887:dbl)
                n670 = Add(x=w864, y=w884) -> (x+y=w883:dbl)
                n671 = Multiply(x=w887, y=0.001) -> (x*y=w874:dbl)
                n672 = Add(x=w880, y=w862) -> (x+y=w879:dbl)
                n673 = Add(x=w882, y=w863) -> (x+y=w881:dbl)
                n674 = global read "Global 1.vi" "ry"() -> (w859:dbl)
                n675 = global read "Global 1.vi" "rz"() -> (w860:dbl)
                n676 = Add(x=w878, y=w861) -> (x+y=w877:dbl)
                n677 = Add(x=w876, y=w859) -> (x+y=w875:dbl)
                n678 = Add(x=w874, y=w860) -> (x+y=w873:dbl)
                n679 = Format Into String(format string="movej( get_inverse_kin(p[%f, %f, %f, %f, %f, %f]), a= 0.5, v=0.25, t=0, r=0)", w883, w881, w879, w877, w875, w873) -> (resulting string=w871:string)  [unwired: 2 in, 1 out]
                n680 = global write "Global 1.vi" "짐빔 카메라 값"(w871) -> ()
                n681 = Wait (ms)(milliseconds to wait=u32 300) -> ()  [unwired: 1 out]
              }
              frame #7 {
                n682 = global write "Global 1.vi" "TCP 스위치"(FALSE ("그리퍼 열림")) -> ()
                n683 = Wait Until Next ms Multiple(millisecond multiple=u32 300 ("milliseconds to wait")) -> ()  [unwired: 1 out]
              }
              frame #8 {
                # "짐빔 위치로 가기"
                n684 = global read "Global 1.vi" "짐빔 카메라 값"() -> (w910:string)
                n685 = invoke class="PrimaryInterfaceScript" method="Send"(reference=w911, "script"=w910) -> (reference out=w908:refnum<k24>)  [unwired: 2 in, 3 out]
                n686 = Wait (ms)(milliseconds to wait=u32 7000) -> ()  [unwired: 1 out]
              }
              frame #9 {
                # "그리퍼 닫기"
                n687 = global write "Global 1.vi" "그리퍼 닫힘"(TRUE ("그리퍼 열림")) -> ()
                n688 = Wait (ms)(milliseconds to wait=u32 300) -> ()  [unwired: 1 out]
              }
              frame #10 {
                n689 = global write "Global 1.vi" "그리퍼 닫힘"(FALSE ("그리퍼 열림")) -> ()
                n690 = Wait (ms)(milliseconds to wait=u32 3000) -> ()  [unwired: 1 out]
              }
              frame #11 {
                # "짐빔 들기"
                n691 = global read "Global 1.vi" "짐빔 들어올리는 자세"() -> (w921:string)
                n692 = invoke class="PrimaryInterfaceScript" method="Send"(reference=w919, "script"=w921) -> (reference out=w918:refnum<k24>)  [unwired: 2 in, 3 out]
                n693 = Wait (ms)(milliseconds to wait=u32 5000) -> ()  [unwired: 1 out]
              }
              frame #12 {
                # "술잔 쪽으로 이동"
                n694 = global read "Global 1.vi" "술잔 위로 가는 자세 2"() -> (w924:string)
                n695 = invoke class="PrimaryInterfaceScript" method="Send"(reference=w923, "script"=w924) -> (reference out=w922:refnum<k24>)  [unwired: 2 in, 3 out]
                n696 = Wait (ms)(milliseconds to wait=u32 15000) -> ()  [unwired: 1 out]
              }
              frame #13 {
                # "술따르기"
                n697 = global read "Global 1.vi" "술 따르는 자세 2"() -> (w927:string)
                n698 = invoke class="PrimaryInterfaceScript" method="Send"(reference=w928, "script"=w927) -> (reference out=w926:refnum<k24>)  [unwired: 2 in, 3 out]
                n699 = Wait (ms)(milliseconds to wait=u32 9000) -> ()  [unwired: 1 out]
              }
              frame #14 {
                # "술따르기 중단"
                n700 = global read "Global 1.vi" "술잔 위로 가는 자세 2"() -> (w932:string)
                n701 = invoke class="PrimaryInterfaceScript" method="Send"(reference=w931, "script"=w932) -> (reference out=w930:refnum<k24>)  [unwired: 2 in, 3 out]
                n702 = Wait (ms)(milliseconds to wait=u32 4000) -> ()  [unwired: 1 out]
              }
              frame #15 {
                # "짐빔 들었던 곳으로"
                n703 = global read "Global 1.vi" "짐빔 들어올리는 자세"() -> (w935:string)
                n704 = invoke class="PrimaryInterfaceScript" method="Send"(reference=w936, "script"=w935) -> (reference out=w934:refnum<k24>)  [unwired: 2 in, 3 out]
                n705 = Wait (ms)(milliseconds to wait=u32 10000) -> ()  [unwired: 1 out]
              }
              frame #16 {
                # "짐빔 내려놓기"
                n706 = global read "Global 1.vi" "짐빔 위치로 가는 자세"() -> (w941:string)
                n707 = invoke class="PrimaryInterfaceScript" method="Send"(reference=w939, "script"=w941) -> (reference out=w938:refnum<k24>)  [unwired: 2 in, 3 out]
                n708 = Wait (ms)(milliseconds to wait=u32 5000) -> ()  [unwired: 1 out]
              }
              frame #17 {
                # "그리퍼 열기"
                n709 = global write "Global 1.vi" "그리퍼 열림"(TRUE ("그리퍼 열림")) -> ()
                n710 = Wait (ms)(milliseconds to wait=u32 300) -> ()  [unwired: 1 out]
              }
              frame #18 {
                n711 = global write "Global 1.vi" "그리퍼 열림"(FALSE ("그리퍼 열림")) -> ()
                n712 = Wait (ms)(milliseconds to wait=u32 3000) -> ()  [unwired: 1 out]
              }
              frame #19 {
                # "짐빔에서 토닉으로 이동준비"
                n713 = global read "Global 1.vi" "짐빔 토닉 이동 준비자세"() -> (w951:string)
                n714 = invoke class="PrimaryInterfaceScript" method="Send"(reference=w949, "script"=w951) -> (reference out=w948:refnum<k24>)  [unwired: 2 in, 3 out]
                n715 = Wait (ms)(milliseconds to wait=u32 5000) -> ()  [unwired: 1 out]
              }
              frame #20 {
                # "토닉보러가기"
                n716 = global read "Global 1.vi" "토닉 보는 자세"() -> (w955:string)
                n717 = invoke class="PrimaryInterfaceScript" method="Send"(reference=w953, "script"=w955) -> (reference out=w952:refnum<k24>)  [unwired: 2 in, 3 out]
                n718 = Wait (ms)(milliseconds to wait=u32 8000) -> ()  [unwired: 1 out]
              }
              frame #21 {
                # "tcp 키는 스위치 보단\n파이썬한테 \n값 보내달라하는\n요청 보내는 걸로 \n바꾸기"
                n719 = global write "Global 1.vi" "몇번 병을 볼것인가"("4" ("몇번 병을 볼것인가")) -> ()
                n720 = global write "Global 1.vi" "TCP 스위치"(TRUE ("그리퍼 열림")) -> ()
                n721 = Wait Until Next ms Multiple(millisecond multiple=u32 500 ("milliseconds to wait")) -> ()  [unwired: 1 out]
              }
              frame #22 {
                n722 = global read "Global 1.vi" "X_부호"() -> (w962:string)
                n723 = global read "Global 1.vi" "Z_부호"() -> (w960:string)
                n724 = global read "Global 1.vi" "Y_부호"() -> (w961:string)
                n725 = case shown="\"1\"" w960 {
                  frame "False", Default {
                  }
                  frame "True" {
                  }
                  frame "2" {
                  }
                  frame "1" {
                    n726 = global read "Global 1.vi" "Z_havetogo"() -> (w968:string)
                    n727 = Decimal String To Number(string=w968) -> (number=w971:i32)  [unwired: 2 in, 1 out]
                    n728 = To Double Precision Float(number=w971) -> (double precision float=w970:dbl)
                    n729 = Format Into String(format string="-%f", w970) -> (resulting string=w967:string)  [unwired: 2 in, 1 out]
                    n730 = global write "Global 1.vi" "Z_havetogo"(w967) -> ()
                  }
                }
                n731 = case shown="\"1\"" w961 {
                  frame "False", Default {
                  }
                  frame "True" {
                  }
                  frame "2" {
                  }
                  frame "1" {
                    n732 = global read "Global 1.vi" "Y_havetogo"() -> (w973:string)
                    n733 = Decimal String To Number(string=w973) -> (number=w976:i32)  [unwired: 2 in, 1 out]
                    n734 = To Double Precision Float(number=w976) -> (double precision float=w974:dbl)
                    n735 = Format Into String(format string="-%f", w974) -> (resulting string=w972:string)  [unwired: 2 in, 1 out]
                    n736 = global write "Global 1.vi" "Y_havetogo"(w972) -> ()
                  }
                }
                n737 = case shown="\"1\"" w962 {
                  frame "False", Default {
                  }
                  frame "True" {
                  }
                  frame "2" {
                  }
                  frame "1" {
                    n738 = global read "Global 1.vi" "X_havetogo"() -> (w978:string)
                    n739 = Decimal String To Number(string=w978) -> (number=w981:i32)  [unwired: 2 in, 1 out]
                    n740 = To Double Precision Float(number=w981) -> (double precision float=w980:dbl)
                    n741 = Format Into String(format string="-%f", w980) -> (resulting string=w977:string)  [unwired: 2 in, 1 out]
                    n742 = global write "Global 1.vi" "X_havetogo"(w977) -> ()
                  }
                }
                n743 = global read "Global 1.vi" "RX_부호"() -> (w965:string)
                n744 = global read "Global 1.vi" "RZ_부호"() -> (w963:string)
                n745 = global read "Global 1.vi" "RY_부호"() -> (w964:string)
                n746 = case shown="\"1\"" w963 {
                  frame "False", Default {
                  }
                  frame "True" {
                  }
                  frame "2" {
                  }
                  frame "1" {
                    n747 = global read "Global 1.vi" "RZ_havetogo"() -> (w983:string)
                    n748 = Decimal String To Number(string=w983) -> (number=w986:i32)  [unwired: 2 in, 1 out]
                    n749 = To Double Precision Float(number=w986) -> (double precision float=w985:dbl)
                    n750 = Format Into String(format string="-%f", w985) -> (resulting string=w982:string)  [unwired: 2 in, 1 out]
                    n751 = global write "Global 1.vi" "RZ_havetogo"(w982) -> ()
                  }
                }
                n752 = case shown="\"1\"" w964 {
                  frame "False", Default {
                  }
                  frame "True" {
                  }
                  frame "2" {
                  }
                  frame "1" {
                    n753 = global read "Global 1.vi" "RY_havetogo"() -> (w988:string)
                    n754 = Decimal String To Number(string=w988) -> (number=w991:i32)  [unwired: 2 in, 1 out]
                    n755 = To Double Precision Float(number=w991) -> (double precision float=w989:dbl)
                    n756 = Format Into String(format string="-%f", w989) -> (resulting string=w987:string)  [unwired: 2 in, 1 out]
                    n757 = global write "Global 1.vi" "RY_havetogo"(w987) -> ()
                  }
                }
                n758 = case shown="\"1\"" w965 {
                  frame "False", Default {
                  }
                  frame "True" {
                  }
                  frame "2" {
                  }
                  frame "1" {
                    n759 = global read "Global 1.vi" "RX_havetogo"() -> (w993:string)
                    n760 = Decimal String To Number(string=w993) -> (number=w996:i32)  [unwired: 2 in, 1 out]
                    n761 = To Double Precision Float(number=w996) -> (double precision float=w995:dbl)
                    n762 = Format Into String(format string="-%f", w995) -> (resulting string=w992:string)  [unwired: 2 in, 1 out]
                    n763 = global write "Global 1.vi" "RX_havetogo"(w992) -> ()
                  }
                }
              }
              frame #23 {
                n764 = global read "Global 1.vi" "X_havetogo"() -> (w1008:string)
                n765 = global read "Global 1.vi" "Y_havetogo"() -> (w1007:string)
                n766 = global read "Global 1.vi" "Z_havetogo"() -> (w1006:string)
                n767 = global read "Global 1.vi" "RX_havetogo"() -> (w1005:string)
                n768 = global read "Global 1.vi" "RY_havetogo"() -> (w1004:string)
                n769 = global read "Global 1.vi" "RZ_havetogo"() -> (w1003:string)
                n770 = Decimal String To Number(string=w1006) -> (number=w1032:i32)  [unwired: 2 in, 1 out]
                n771 = Decimal String To Number(string=w1008) -> (number=w1038:i32)  [unwired: 2 in, 1 out]
                n772 = Decimal String To Number(string=w1007) -> (number=w1035:i32)  [unwired: 2 in, 1 out]
                n773 = Decimal String To Number(string=w1005) -> (number=w1029:i32)  [unwired: 2 in, 1 out]
                n774 = Decimal String To Number(string=w1004) -> (number=w1026:i32)  [unwired: 2 in, 1 out]
                n775 = Decimal String To Number(string=w1003) -> (number=w1023:i32)  [unwired: 2 in, 1 out]
                n776 = To Double Precision Float(number=w1032) -> (double precision float=w1034:dbl)
                n777 = To Double Precision Float(number=w1038) -> (double precision float=w1040:dbl)
                n778 = To Double Precision Float(number=w1035) -> (double precision float=w1037:dbl)
                n779 = To Double Precision Float(number=w1029) -> (double precision float=w1031:dbl)
                n780 = To Double Precision Float(number=w1026) -> (double precision float=w1028:dbl)
                n781 = Multiply(x=w1040, y=0.001) -> (x*y=w1022:dbl)
                n782 = Multiply(x=w1034, y=0.001) -> (x*y=w1018:dbl)
                n783 = Multiply(x=w1037, y=0.001) -> (x*y=w1020:dbl)
                n784 = Multiply(x=w1031, y=0.001) -> (x*y=w1016:dbl)
                n785 = global read "Global 1.vi" "x"() -> (w1002:dbl)
                n786 = Multiply(x=w1028, y=0.001) -> (x*y=w1014:dbl)
                n787 = global read "Global 1.vi" "y"() -> (w1001:dbl)
                n788 = global read "Global 1.vi" "rx"() -> (w999:dbl)
                n789 = global read "Global 1.vi" "z"() -> (w1000:dbl)
                n790 = To Double Precision Float(number=w1023) -> (double precision float=w1025:dbl)
                n791 = Add(x=w1002, y=w1022) -> (x+y=w1021:dbl)
                n792 = Multiply(x=w1025, y=0.001) -> (x*y=w1012:dbl)
                n793 = Add(x=w1018, y=w1000) -> (x+y=w1017:dbl)
                n794 = Add(x=w1020, y=w1001) -> (x+y=w1019:dbl)
                n795 = global read "Global 1.vi" "ry"() -> (w997:dbl)
                n796 = global read "Global 1.vi" "rz"() -> (w998:dbl)
                n797 = Add(x=w1016, y=w999) -> (x+y=w1015:dbl)
                n798 = Add(x=w1014, y=w997) -> (x+y=w1013:dbl)
                n799 = Add(x=w1012, y=w998) -> (x+y=w1011:dbl)
                n800 = Format Into String(format string="movej( get_inverse_kin(p[%f, %f, %f, %f, %f, %f]), a= 0.5, v=0.25, t=0, r=0)", w1021, w1019, w1017, w1015, w1013, w1011) -> (resulting string=w1009:string)  [unwired: 2 in, 1 out]
                n801 = global write "Global 1.vi" "토닉 카메라 값"(w1009) -> ()
                n802 = Wait (ms)(milliseconds to wait=u32 300) -> ()  [unwired: 1 out]
              }
              frame #24 {
                n803 = global write "Global 1.vi" "TCP 스위치"(FALSE ("그리퍼 열림")) -> ()
                n804 = Wait Until Next ms Multiple(millisecond multiple=u32 300 ("milliseconds to wait")) -> ()  [unwired: 1 out]
              }
              frame #25 {
                # "토닉 들러가기"
                n805 = global read "Global 1.vi" "토닉 카메라 값"() -> (w1049:string)
                n806 = invoke class="PrimaryInterfaceScript" method="Send"(reference=w1047, "script"=w1049) -> (reference out=w1046:refnum<k24>)  [unwired: 2 in, 3 out]
                n807 = Wait (ms)(milliseconds to wait=u32 8000) -> ()  [unwired: 1 out]
              }
              frame #26 {
                n808 = global write "Global 1.vi" "그리퍼 닫힘"(TRUE ("그리퍼 열림")) -> ()
                n809 = Wait (ms)(milliseconds to wait=u32 300) -> ()  [unwired: 1 out]
              }
              frame #27 {
                n810 = global write "Global 1.vi" "그리퍼 닫힘"(FALSE ("그리퍼 열림")) -> ()
                n811 = Wait (ms)(milliseconds to wait=u32 3000) -> ()  [unwired: 1 out]
              }
              frame #28 {
                # "토닉 들어올리기"
                n812 = global read "Global 1.vi" "토닉 드는 자세"() -> (w1059:string)
                n813 = invoke class="PrimaryInterfaceScript" method="Send"(reference=w1057, "script"=w1059) -> (reference out=w1056:refnum<k24>)  [unwired: 2 in, 3 out]
                n814 = Wait (ms)(milliseconds to wait=u32 5000) -> ()  [unwired: 1 out]
              }
              frame #29 {
                # "토닉 살짝 빼기"
                n815 = global read "Global 1.vi" "토닉 빼는 자세"() -> (w1063:string)
                n816 = invoke class="PrimaryInterfaceScript" method="Send"(reference=w1061, "script"=w1063) -> (reference out=w1060:refnum<k24>)  [unwired: 2 in, 3 out]
                n817 = Wait (ms)(milliseconds to wait=u32 7000) -> ()  [unwired: 1 out]
              }
              frame #30 {
                # "술잔으로 이동"
                n818 = global read "Global 1.vi" "술잔 위로 가는 자세 2"() -> (w1067:string)
                n819 = invoke class="PrimaryInterfaceScript" method="Send"(reference=w1065, "script"=w1067) -> (reference out=w1064:refnum<k24>)  [unwired: 2 in, 3 out]
                n820 = Wait (ms)(milliseconds to wait=u32 12000) -> ()  [unwired: 1 out]
              }
              frame #31 {
                # "술잔에 따르기"
                n821 = global read "Global 1.vi" "술 따르는 자세 2"() -> (w1071:string)
                n822 = invoke class="PrimaryInterfaceScript" method="Send"(reference=w1069, "script"=w1071) -> (reference out=w1068:refnum<k24>)  [unwired: 2 in, 3 out]
                n823 = Wait (ms)(milliseconds to wait=u32 13000) -> ()  [unwired: 1 out]
              }
              frame #32 {
                # "술따르기 중단"
                n824 = global read "Global 1.vi" "술잔 위로 가는 자세 2"() -> (w1075:string)
                n825 = invoke class="PrimaryInterfaceScript" method="Send"(reference=w1073, "script"=w1075) -> (reference out=w1072:refnum<k24>)  [unwired: 2 in, 3 out]
                n826 = Wait (ms)(milliseconds to wait=u32 5000) -> ()  [unwired: 1 out]
              }
              frame #33 {
                # "토닉 뻇던 자세로 복귀"
                n827 = global read "Global 1.vi" "토닉 빼는 자세"() -> (w1078:string)
                n828 = invoke class="PrimaryInterfaceScript" method="Send"(reference=w1077, "script"=w1078) -> (reference out=w1076:refnum<k24>)  [unwired: 2 in, 3 out]
                n829 = Wait (ms)(milliseconds to wait=u32 9000) -> ()  [unwired: 1 out]
              }
              frame #34 {
                # "토닉 내려놓으러 가기"
                n830 = global read "Global 1.vi" "토닉 드는 자세"() -> (w1083:string)
                n831 = invoke class="PrimaryInterfaceScript" method="Send"(reference=w1081, "script"=w1083) -> (reference out=w1080:refnum<k24>)  [unwired: 2 in, 3 out]
                n832 = Wait (ms)(milliseconds to wait=u32 7000) -> ()  [unwired: 1 out]
              }
              frame #35 {
                # "토닉 내려놓기"
                n833 = global read "Global 1.vi" "토닉 가는자세"() -> (w1087:string)
                n834 = invoke class="PrimaryInterfaceScript" method="Send"(reference=w1085, "script"=w1087) -> (reference out=w1084:refnum<k24>)  [unwired: 2 in, 3 out]
                n835 = Wait (ms)(milliseconds to wait=u32 5000) -> ()  [unwired: 1 out]
              }
              frame #36 {
                # "그리퍼 열기"
                n836 = global write "Global 1.vi" "그리퍼 열림"(TRUE ("그리퍼 열림")) -> ()
                n837 = Wait (ms)(milliseconds to wait=u32 300) -> ()  [unwired: 1 out]
              }
              frame #37 {
                n838 = global write "Global 1.vi" "그리퍼 열림"(FALSE ("그리퍼 열림")) -> ()
                n839 = Wait (ms)(milliseconds to wait=u32 3000) -> ()  [unwired: 1 out]
              }
              frame #38 {
                # "토닉 뻇던 자세로 복귀"
                n840 = global read "Global 1.vi" "토닉 빼는 자세"() -> (w1096:string)
                n841 = invoke class="PrimaryInterfaceScript" method="Send"(reference=w1095, "script"=w1096) -> (reference out=w1094:refnum<k24>)  [unwired: 2 in, 3 out]
                n842 = Wait (ms)(milliseconds to wait=u32 5000) -> ()  [unwired: 1 out]
              }
              frame #39 {
                # "초기자세"
                n843 = global read "Global 1.vi" "1자로 서는 자세"() -> (w1100:string)
                n844 = invoke class="PrimaryInterfaceScript" method="Send"(reference=w1098, "script"=w1100) -> ()  [unwired: 2 in, 4 out]
                n845 = Wait (ms)(milliseconds to wait=u32 15000) -> ()  [unwired: 1 out]
              }
              frame #40 {
                n846 = global write "Global 1.vi" "그리퍼 닫힘"(TRUE ("그리퍼 열림")) -> ()
                n847 = Wait (ms)(milliseconds to wait=u32 300) -> ()  [unwired: 1 out]
              }
              frame #41 {
                w1103 = ""
                # "그리퍼의 앙다문 일자 입"
                n848 = global write "Global 1.vi" "그리퍼 닫힘"(FALSE ("그리퍼 열림")) -> ()
                n849 = Wait (ms)(milliseconds to wait=u32 3000) -> ()  [unwired: 1 out]
                n850 = global write "Global 1.vi" "잭다니엘 카메라 값"(w1103) -> ()
                n851 = global write "Global 1.vi" "콜라 카메라 값"(w1103) -> ()
                n852 = global write "Global 1.vi" "토닉 카메라 값"(w1103) -> ()
                n853 = global write "Global 1.vi" "짐빔 카메라 값"(w1103) -> ()
              }
            }
          }
          frame 5 {
            # "multi order"
          }
          frame 6 {
            # "multi order"
          }
          frame 7 {
            # "multi order"
          }
        }
        n854 = case shown="True" "Send script" {
          tunnel: w51 -> [_ w1112]
          frame False {
          }
          frame True {
            n855 = flat-sequence {
              tunnel: w1112 -> [w1114]
              frame #0 {
                n856 = invoke class="PrimaryInterfaceScript" method="Send"(reference=w1114, "script"="Script to execute") -> ()  [unwired: 2 in, 4 out]
              }
            }
          }
        }
        n857 = case shown="True" "Move to Zero position" {
          tunnel: w51 -> [_ w1109]
          frame False {
          }
          frame True {
            n858 = flat-sequence {
              tunnel: w1109 -> [w1111]
              frame #0 {
                n859 = invoke class="PrimaryInterfaceScript" method="Send"(reference=w1111, "script"="movej([3.1412,-1.5708,0,-1.5708,3.1412,5.8904], a=0.5, v=0.25, t=0, r=0)") -> ()  [unwired: 2 in, 4 out]
              }
            }
          }
        }
        n860 = case shown="True" "Move to particular posture" {
          tunnel: w51 -> [_ w1106]
          frame False {
          }
          frame True {
            n861 = flat-sequence {
              tunnel: w1106 -> [w1108]
              frame #0 {
                n862 = invoke class="PrimaryInterfaceScript" method="Send"(reference=w1108, "script"="movej([-1.5,-1.5,-2,-0.5,1.8,0], a=1.4, v=1.05, t=0, r=0)") -> ()  [unwired: 2 in, 4 out]
              }
            }
          }
        }
        n863 = property class="PrimaryInterfaceClientInternal"(reference=w50) -> ("RobotModeData"=w63:refnum<k24>)  [unwired: 1 in, 2 out]
        n864 = property class="PrimaryInterfaceClientInternal"(reference=w50) -> ("CartesianInfo"=w49:refnum<k24>)  [unwired: 1 in, 2 out]
        n865 = property class="RobotModeDataPackageEventArgs"(reference=w63) -> ("RobotPowerOn"=→"Powered on":bool)  [unwired: 1 in, 2 out]
        n866 = constructor class="SocketCommunicationServer"() -> (reference out=w59:refnum<k24>)  [unwired: 3 in, 2 out]
        n867 = property class="SocketCommunicationServer"(reference=w59) -> ("Enabled"=→"Enabled":bool)  [unwired: 1 in, 2 out]
        n868 = property class="SocketCommunicationServer"(reference=w59) -> ("Port"=→"Port":i32)  [unwired: 1 in, 2 out]
        n869 = property class="CartesianInfoPackageEventArgs"(reference=w49) -> ("Y"=→"Y":dbl)  [unwired: 1 in, 2 out]
        n870 = property class="CartesianInfoPackageEventArgs"(reference=w49) -> ("Ry"=→"Ry":dbl)  [unwired: 1 in, 2 out]
        n871 = property class="CartesianInfoPackageEventArgs"(reference=w49) -> ("Z"=→"Z":dbl)  [unwired: 1 in, 2 out]
        n872 = property class="CartesianInfoPackageEventArgs"(reference=w49) -> ("Rz"=→"Rz":dbl)  [unwired: 1 in, 2 out]
        n873 = property class="CartesianInfoPackageEventArgs"(reference=w49) -> ("X"=→"X":dbl)  [unwired: 1 in, 2 out]
        n874 = property class="CartesianInfoPackageEventArgs"(reference=w49) -> ("Rx"=→"Rx":dbl)  [unwired: 1 in, 2 out]
      }
    }
    n875 = property class="UR"(reference=w34) -> ("Dashboard"=w38:refnum<k24>)  [unwired: 1 in, 2 out]
    n876 = case shown="True" "Power off" {
      tunnel: w38 -> [_ w1115]
      frame False {
      }
      frame True {
        n877 = flat-sequence {
          tunnel: w1115 -> [w1116]
          frame #0 {
            n878 = invoke class="DashboardClientInternal" method="PowerOff"(reference=w1116) -> ()  [unwired: 2 in, 3 out]
          }
        }
      }
    }
    n879 = case shown="True" "Power on\nRelease brake" {
      tunnel: w38 -> [_ w1117]
      frame False {
      }
      frame True {
        n880 = flat-sequence {
          tunnel: w1117 -> [w1119]
          frame #0 {
            n881 = invoke class="DashboardClientInternal" method="PowerOn"(reference=w1119) -> (reference out=w1118:refnum<k24>)  [unwired: 2 in, 2 out]
            n882 = invoke class="DashboardClientInternal" method="ReleaseBrake"(reference=w1118) -> ()  [unwired: 2 in, 3 out]
          }
        }
      }
    }
  }
  n883 = invoke class="UR" method="RegisterLicense"(reference=w28, "licensee"="your company name", "key"="") -> (reference out=w30:refnum<k24>)  [unwired: 2 in, 4 out]
  n884 = control-ref of="Script to execute"() -> (w27:refnum<vi>)
  n885 = property class="Str"(reference=w27, "Value"="movej([-1.5,-1.5,-2,-0.5,1.8,0], a=1.4, v=1.05, t=0, r=0)") -> ()  [unwired: 1 in, 2 out]
  n886 = property class="UR"(reference=w30) -> ("LicenseInfo"=w29:refnum<k24>)  [unwired: 1 in, 2 out]
  n887 = invoke class="LicenseInfo" method="ToString"(reference=w29) -> ("ToString"=→"License state":string)  [unwired: 2 in, 2 out]
  n888 = global read "Global 1.vi" "TCP 스위치"() -> (w1:bool)
  n889 = case shown="True" w1 {
    frame False {
      w1124 = "0"
      n890 = global write "Global 1.vi" "지호씨가 보낸 총 좌표"(w1124) -> ()
      n891 = global write "Global 1.vi" "RY_havetogo"(w1124) -> ()
      n892 = global write "Global 1.vi" "RZ_havetogo"(w1124) -> ()
      n893 = global write "Global 1.vi" "RX_havetogo"(w1124) -> ()
      n894 = global write "Global 1.vi" "Y_havetogo"(w1124) -> ()
      n895 = global write "Global 1.vi" "Z_havetogo"(w1124) -> ()
      n896 = global write "Global 1.vi" "X_havetogo"(w1124) -> ()
      n897 = global write "Global 1.vi" "RY_부호"(w1124) -> ()
      n898 = global write "Global 1.vi" "RZ_부호"(w1124) -> ()
      n899 = global write "Global 1.vi" "RX_부호"(w1124) -> ()
      n900 = global write "Global 1.vi" "Y_부호"(w1124) -> ()
      n901 = global write "Global 1.vi" "Z_부호"(w1124) -> ()
      n902 = global write "Global 1.vi" "X_부호"(w1124) -> ()
    }
    frame True {
      w1161 = 4 ("length (rest)")
      n903 = global read "Global 1.vi" "몇번 병을 볼것인가"() -> (w1152:string)
      n904 = TCP Open Connection(address="192.168.112.18", remote port or service name=u16 8089) -> (connection ID=w1156:refnum<k5>, error out=w1155:errorcluster)  [unwired: 3 in]
      n905 = TCP Write(connection ID=w1156, data in=w1152, error in (no error)=w1155) -> (connection ID out=w1154:refnum<k5>, error out=w1153:errorcluster)  [unwired: 1 in, 1 out]
      n906 = TCP Read(connection ID=w1154, bytes to read=30, error in (no error)=w1153, 7:T1."Buffered" ("mode (standard)")) -> (connection ID out=w1165:refnum<k5>, data out=w1125:string, error out=w1164:errorcluster)  [unwired: 1 in]
      n907 = String Subset(string=w1125, offset (0)=11, length (rest)=w1161) -> (substring=w1143:string)
      n908 = String Subset(string=w1125, offset (0)=16, length (rest)=w1161) -> (substring=w1142:string)
      n909 = String Subset(string=w1125, offset (0)=6, length (rest)=w1161) -> (substring=w1144:string)
      n910 = String Subset(string=w1125, offset (0)=1, length (rest)=w1161) -> (substring=w1145:string)
      n911 = global write "Global 1.vi" "X_havetogo"(w1145) -> ()
      n912 = global write "Global 1.vi" "Z_havetogo"(w1143) -> ()
      n913 = global write "Global 1.vi" "RX_havetogo"(w1142) -> ()
      n914 = global write "Global 1.vi" "Y_havetogo"(w1144) -> ()
      n915 = String Subset(string=w1125, offset (0)=26, length (rest)=w1161) -> (substring=w1140:string)
      n916 = String Subset(string=w1125, offset (0)=21, length (rest)=w1161) -> (substring=w1141:string)
      n917 = global write "Global 1.vi" "지호씨가 보낸 총 좌표"(w1125) -> ()
      n918 = String Subset(string=w1125, offset (0)=20, length (rest)=1 ("length (rest)")) -> (substring=w1138:string)
      n919 = String Subset(string=w1125, offset (0)=15, length (rest)=1 ("length (rest)")) -> (substring=w1139:string)
      n920 = String Subset(string=w1125, offset (0)=25, length (rest)=1 ("length (rest)")) -> (substring=w1137:string)
      n921 = global write "Global 1.vi" "RY_havetogo"(w1141) -> ()
      n922 = TCP Close Connection(connection ID=w1165, error in (no error)=w1164) -> ()  [unwired: 1 in, 2 out]
      n923 = global write "Global 1.vi" "RZ_havetogo"(w1140) -> ()
      n924 = global write "Global 1.vi" "RY_부호"(w1138) -> ()
      n925 = global write "Global 1.vi" "RX_부호"(w1139) -> ()
      n926 = global write "Global 1.vi" "RZ_부호"(w1137) -> ()
      n927 = String Subset(string=w1125, offset (0)=0, length (rest)=1 ("length (rest)")) -> (substring=w1134:string)
      n928 = String Subset(string=w1125, offset (0)=5, length (rest)=1 ("length (rest)")) -> (substring=w1131:string)
      n929 = String Subset(string=w1125, offset (0)=10, length (rest)=1 ("length (rest)")) -> (substring=w1128:string)
      n930 = global write "Global 1.vi" "X_부호"(w1134) -> ()
      n931 = global write "Global 1.vi" "Y_부호"(w1131) -> ()
      n932 = global write "Global 1.vi" "Z_부호"(w1128) -> ()
    }
  }
